vi "FocalMainWakeStudyV3.vi"() -> ()   [LabVIEW 2018]
uses:
  Clusters/FileDataChannel.ctl
  Clusters/BladePitchMode.ctl
  Clusters/GenMode.ctl
  Clusters/IndicatorScale.ctl
  Clusters/SimulationConstants.ctl
  Clusters/PLCTravSignals.ctl
  Clusters/IOSignals.ctl
  <vilib>/Platform/TimedLoop/XDataNode/timing_clust.ctl
  <vilib>/Platform/TimedLoop/XDataNode/nitl_modes.ctl
  <vilib>/Platform/TimedLoop/XDataNode/wakeup.ctl
  Clusters/ArrayPairs.ctl
  Clusters/SwapArrayCluster.ctl
  Clusters/ElmoState.ctl
  Clusters/CtrlSignals.ctl
  Clusters/ScalingEnum.ctl
  Clusters/AnemometerData.ctl
  Clusters/RoscoParams.ctl
  Clusters/GenCtrl.ctl
  Clusters/PitchCtrl.ctl
  <vilib>/Instr/_visa.llb/VISA Configure Serial Port (Instr).vi
  SubVIs/InsertIntoArray_v2.vi
  <vilib>/platform/TimedLoop/XDataNode/XDataNode.xnode
  <vilib>/Platform/TimedLoop/XDataNode/XDNodeRunTimeDep.lvlib
  <resource>/objmgr/IndComECAT.rc
  usr/local/lib/libCallROSCO.so
  <vilib>/ptbypt/NI_PtbyPt.lvlib
panel:
  out "anemoXprobeD2_m_s":dbl
  out "anemoXprobeD1_m_s":dbl
  out "anemoXprobeC2_m_s":dbl
  out "anemoXprobeC1_m_s":dbl
  out "traversePosZ_mm":dbl
  out "traversePosY_mm":dbl
  out "traversePosX_mm":dbl
  in  "PLCTravSignals":T1
  out "WE ROSCO":dbl
  out "Mz":dbl format="%#_5g"
  out "My":dbl format="%#_5g"
  out "Mx":dbl format="%#_5g"
  in  "zeroRotorPos":bool
  out "Fz":dbl format="%#_5g"
  out "TSR":dbl
  out "anemoRefU_m_s":dbl
  out "RS232 loop late?":bool
  in  "Fan Setpoint (%)":dbl format="%#_13g"
  out "Setpoint file loaded":path
  in  "Ctrl Mode":enum32{"Manual", "FromFile"}(radio)
  in  "Setpoint file name":string="setpointsVelTestA.txt"
  in  "Reload File":bool
  in  "windSpeed_m_s":dbl format="%#_13g"
  out "towerBotMy":dbl
  out "Current Setting":dbl[](array[numeric])
  in  "Commit":bool
  in  "Clear Faults":bool
  in  "Enable Fans":bool
  in  "Turn Fans On":bool
  out "Fy":dbl format="%#_5g"
  out "Fx":dbl
  out "PLC read errors":string
  out "PLC read/write late?":bool
  out "PLC Read Error":bool
  out "Axis 3 Homing":bool
  out "Axis 2 Homing":bool
  out "Axis 1 Homing":bool
  in  "Home Blades (x3)":bool
  out "Axis 3 Homed":bool
  out "Axis 2 Homed":bool
  out "Axis 1 Homed":bool
  out "SimulationConst":T2={"nGear"=1.0, "rotorRadius"=120.0, "numBlades"=3, "scaleFactor"=70.0, "roscoInitMinSpeed_rad_s"=0.5, "roscoInitMinTorqueFS_Nm"=1000000.0, "beckhoff16bit"=1000000.0, "beckhoff24BitExt"=7812500, "BX824Bit"=0, "rotorTorqueScale_Nm_V"=5.0, "rotorTorqueOfst_Nm"=2.0, "rangeEL3104V"=10.0, "nacelleAccELM3604V"=1.25, "nacelleAccScaleX_m_s2_V"=0.0673, "nacelleAccOfstX_m_s2"=0.0055, "nacelleAccScaleY_m_s2_V"=0.0672, "nacelleAccOfstY_m_s2"=0.0049, "nacelleAccScaleZ_m_s2_V"=0.0677, "nacelleAccOfstZ_m_s2"=0.0087, "cyberGearRatio"=0.5, "cyberLinesPerRev"=0.5, "cyberRatedTorque"=0.5, "towerTopForceScale"=0.5, "towerTopTorqueScale"=0.5, "plcSetpointScaling_norm2VFD"=0.5, "towerBotScaleMy_Nm_V"=0.5, "towerBotOfstMy_Nm"=0.5, "towerTopScaleXaxis_N_V"=0.5, "towerTopOfstXaxis_N"=0.5, "towerTopScaleYaxis_N_V"=0.5, "towerTopOfstYaxis_N"=0.5, "pitchFlagOffset_deg"=0.5, "anemWindSpeedScaleU_m_s_m_s"=0.5, "anemWindSpeedOfstU_m_s"=0.5, "anemWindSpeedScaleV_m_s_m_s"=0.5, "anemWindSpeedOfstV_m_s"=0.5, "anemWindSpeedScaleW_m_s_m_s"=0.5, "anemWindSpeedOfstW_m_s"=0.5, "anemWindSpeedScaleTSI1_m_s_V"=0.5, "anemWindSpeedOfstTSI1_m_s"=0.5, "anemWindSpeedScaleTSI3_m_s_V"=0.5, "anemWindSpeedOfstTSI3_m_s"=0.5, "anemWindSpeedScaleXProbeA1C0"=0.5, "anemWindSpeedScaleXProbeA1C1"=0.5, "anemWindSpeedScaleXProbeA1C2"=0.5, "anemWindSpeedScaleXProbeA1C3"=0.5, "anemWindSpeedScaleXProbeA1C4"=0.5, "anemWindSpeedOfstXProbeA1_m_s"=0.5, "anemWindSpeedScaleXProbeA2C0"=0.5, "anemWindSpeedScaleXProbeA2C1"=0.5, "anemWindSpeedScaleXProbeA2C2"=0.5, "anemWindSpeedScaleXProbeA2C3"=0.5, "anemWindSpeedScaleXProbeA2C4"=0.5, "anemWindSpeedOfstXProbeA2_m_s"=0.5, "anemWindSpeedScaleXProbeC1C0"=0.5, "anemWindSpeedScaleXProbeC1C1"=0.5, "anemWindSpeedScaleXProbeC1C2"=0.5, "anemWindSpeedScaleXProbeC1C3"=0.5, "anemWindSpeedScaleXProbeC1C4"=0.5, "anemWindSpeedOfstXProbeC1_m_s"=0.5, "anemWindSpeedScaleXProbeC2C0"=0.5, "anemWindSpeedScaleXProbeC2C1"=0.5, "anemWindSpeedScaleXProbeC2C2"=0.5, "anemWindSpeedScaleXProbeC2C3"=0.5, "anemWindSpeedScaleXProbeC2C4"=0.5, "anemWindSpeedOfstXProbeC2_m_s"=0.5, "anemWindSpeedScaleXProbeD1C0"=0.5, "anemWindSpeedScaleXProbeD1C1"=0.5, "anemWindSpeedScaleXProbeD1C2"=0.5, "anemWindSpeedScaleXProbeD1C3"=0.5, "anemWindSpeedScaleXProbeD1C4"=0.5, "anemWindSpeedOfstXProbeD1_m_s"=0.5, "anemWindSpeedScaleXProbeD2C0"=0.5, "anemWindSpeedScaleXProbeD2C1"=0.5, "anemWindSpeedScaleXProbeD2C2"=0.5, "anemWindSpeedScaleXProbeD2C3"=0.5, "anemWindSpeedScaleXProbeD2C4"=0.5, "anemWindSpeedOfstXProbeD2_m_s"=0.5, "anemWindSpeedOfstHw3_m_s"=0.5, "anemWindSpeedScaleHw3_m_s_V"=0.5, "probeAOfstX_mm"=0.5, "probeAOfstY_mm"=0.5, "probeAOfstZ_mm"=0.5, "probeTSIOfstX_mm"=0.5, "probeTSIOfstY_mm"=0.5, "probeTSIOfstZ_mm"=0.5, "probeBOfstX_mm"=0.5, "probeBOfstY_mm"=0.5, "probeBOfstZ_mm"=0.5} {"beckhoff16bit" format="%x"}
  out "nacelleAccZ (m/s2)":dbl
  out "nacelleAccY (m/s2)":dbl
  out "nacelleAccX (m/s2)":dbl
  out "Disk > 2GB free?":bool
  out "Current OP mode":T3
  in  "IndicatorScale":T4
  in  "DISCON.IN file":string="IEA15MW_FOCAL_04_DISCON.IN"
  in  "Cp/Ct/Cq file":string="IEA15MW_FOCAL_00_Cp_Ct_Cq.txt"
  out "Torque sine period FS (Nm)":dbl format="%.2g"
  out "Torque sine amp FS (Nm)":dbl format="%.2g"
  out "Torque sine mean FS (Nm)":dbl format="%.2g"
  out "Ramp time FS (s)":dbl format="%.2g"
  out "Ramp target vel FS (rpm)":dbl format="%.2g"
  out "Const. vel setpoint FS (rpm)":dbl format="%.2g"
  out "From File RotSpd FS (rpm)":dbl
  out "From File Pitch FS (deg)":dbl
  out "Exp time FS (s)":dbl format="%5.2f"
  in  "Commit gen settings":bool
  out "Current OP mode":T5
  in  "Commit pitch settings":bool
  in  "Start / Stop Run":bool
  out "Speed Setpoint (rpm)":dbl(knob)=7.068579725455493e-05 scale=0.0..20.0
  out "Pitch Blade 3 (deg)":dbl
  out "Pitch Bade 2 (deg)":dbl
  out "Pitch Blade 1 (deg)":dbl
  out "Pitch Setpoint (deg)":dbl
  out "Torque sine period MS (Nm)":dbl format="%.2g"
  out "Torque sine amp MS (Nm)":dbl format="%#.2g"
  in  "Torque sine period (s)":dbl=100.0
  in  "Torque sine amp (MNm)":dbl
  out "Torque sine mean MS (Nm)":dbl format="%.2g"
  in  "Torque mean (MNm)":dbl
  out "Ramp time MS (s)":dbl format="%.2g"
  out "Ramp target vel MS (rpm)":dbl format="%.2g"
  out "Const. vel setpoint MS (rpm)":dbl format="%.2g"
  in  "Ramp time (s)":dbl=100.0
  in  "Ramp target vel (rpm)":dbl=1.0
  in  "Const. vel (rpm)":dbl
  out "Current Const. (deg)":dbl
  in  "Next OP mode":T3
  in  "Next Const. (deg)":dbl=10.0
  in  "Next OP mode":T5
  in  "Wind Est. u(t=0)":dbl=5.0
  out "Exp. Time MS (s)":dbl format="%5.1f"
  out "Output file Name":string
  out "State logic late?":bool
  out "Axis 3 Fault":bool
  out "Axis 3 Warning":bool
  out "Axis 2 Fault":bool
  out "Axis 2 Warning":bool
  out "Axis 1 Fault":bool
  out "Axis 1 Warning":bool
  out "Axis 3 Operational":bool
  out "Axis 2 Operational":bool
  out "Axis 1 Operational":bool
  out "Pitch Axis 3 State":string
  out "Pitch Axis 2 State":string
  out "Pitch Axis 1 State":string
  in  "Clear Pitch Actuator Faults (x3)":bool
  in  "Enable Pitch Actuators (x3)":bool
  out "Generator Operational":bool
  in  "Clear Accelnet Faults":bool
  in  "Enable Accelnet":bool
  out "Generator Fault":bool
  out "Generator Warning":bool
  out "Main generator state":string
  out "Rosco Failed?":bool
  out "Torque Cell":dbl(knob) scale=0.0..25.0
  out "Actual Speed MS (rpm)":dbl(knob)=7.068579725455493e-05 scale=0.0..20.0
  in  "?":T6(tab)
  out "Generator Speed":dynamicdata(graph)
  out "Rotor Loads":dynamicdata(graph)
  out "Pitch":dynamicdata(graph)
  in  "Sample":bool
  in  "Apply Ofst":bool
  out "FxMean":dbl format="%0.2f"
  out "FyMean":dbl format="%0.2f"
  out "FzMean":dbl format="%0.2f"
  out "MxMean":dbl format="%0.2f"
  out "MyMean":dbl format="%0.2f"
  out "MzMean":dbl format="%0.2f"
  out "botMyMean":dbl format="%0.2f"
  out "pitch1_deg":dbl
  out "pitch2_deg":dbl
  out "pitch3_deg":dbl
  in  "pitch1 Ofst (deg)":dbl
  in  "pitch3 Ofst (deg)":dbl=-1.5
  in  "pitch2 Ofst (deg)":dbl
  out "Wind":dynamicdata(graph)
  out "DISCON.IN Contents":string
  out "Rosco Interface Current Message":string
  out "ROSCO DISCON.In file used":string
  out "ROSCO CpCqCt File used":string
  out "ROSCO out file used":string
  out "Test sum":sgl
  out "error out":errorcluster
  out "aviFAIL":i32
  out "Rosco Interface First Message":string
  out "Rosco Setpoint (Nm) - MS":dbl(knob) scale=0.0..10.0
  out "OUT_ROTSP":dbl
  out "OUT_AEROTQ":dbl
  out "Rosco Pitch Setpoint (rad)":dbl(knob) scale=0.0..10.0
  out "avrSWAP":dbl[](array[numeric])
  out "Setpoints":dbl[][](array[numeric])
  out "Time index":i32
  out "Loop duration (ms)":i64
  in  "Pitch Max Vel Change (rpm/min) - FS":dbl=10.0
  in  "Pitch Max Vel (rpm) - FS":dbl=1.0
  in  "Pitch Homing Vel  (rpm) - FS":dbl=0.3
  in  "Pitch P-Gain":dbl=5.0
  in  "Max Vel (rpm)  -FS":dbl=14.0
  in  "Velocity Ctrl P-Gain":dbl=0.14
  in  "Velocity Ctrl I-Gain":dbl=3.0
  in  "Torque Ctrl FF Gain":dbl=0.35
  in  "Torque Ctrl I-Gain":dbl=12.5
  in  "Torque Ctrl P-Gain":dbl=0.3
  in  "Max Torque (MNm) - FS":dbl=25.0
  out "Pitch axis 3 ctrl word":u16 format="%x"
  out "Pitch axis 2 ctrl word":u16 format="%x"
  out "RT Loop Duration":i64
  out "Control Mode - Main Gen":u8
  out "WriteSDO Abort - Main Gen":u32
  out "ReadSDO Abort - Main Gen":u32
  out "Gen ctrl word":u16 format="%x"
  out "Pitch axis 1 ctrl word":u16 format="%x"
  out "Graphics Update t (s)":dbl format="%.1f"
  out "Effective graphics rate (ms)":dbl format="%#.1f"
  out "WriteSDO Abort - Pitch 1":u32
  out "ReadSDO Abort - Pitch 1":u32
  out "Control Mode - Pitch 1":u8
  out "Torque RAW (V)":dbl
  out "Torque Sensor (Nm) - NOT scaled":dbl(knob) scale=-2.0..2.0
  out "Free GB disk":dbl
  out "WriteSDO Abort - Pitch 2":u32
  out "Control Mode - Pitch 2":u8
  out "ReadSDO Abort - Pitch 2":u32
  out "WriteSDO Abort - Pitch 3":u32
  out "Control Mode - Pitch 3":u8
  out "ReadSDO Abort - Pitch 3":u32
  out "MotorDemandTorque_Nm":dbl(knob) scale=-2.0..2.0
  out "MotorCurrentTorq (Nm)":dbl(knob) scale=-2.0..2.0
  out "Axis 1 HomePos (rad)":dbl
  out "Axis 2 HomePos (rad)":dbl
  out "Axis 3 HomePos (rad)":dbl
  out "mainGenPosition (deg)":dbl
  out "Init error":errorcluster
  out "Setpoint read error":string
  out "ROSCO Tq Setpoint":dbl(knob) scale=0.0..35.0
  out "Power (MW)":dbl(slide) scale=0.0..30.0 scale format="%.2f"
  out "FIFO Loop Late?":bool
  in  "Base filename":string="rosco-tests"
  out "Writing":bool
  in  "?":T7
  out "#RT FIFO":u32
  in  "Stop LabVIEW":bool
  out "cRio Time(s)":dbl format="%6.1f"
  out "RT Loop Late?":bool
  # "FOCAL Campaign 1 - V2.1"
  # "ROSCO OK?"
  # "GENERATOR ENABLE"
  # "BLADE PITCH"
  # "WIND MACHINE CONTROL"
  # "EXPERIMENT CONTROL"
  # "GENERATOR SETPOINT CTRL"
  # "PITCH ACTUATORS CONTROL"
  # "Nacelle Acceleration"
  # "TowerTop 6DOF"
  # "Blade1"
  # "Blade2"
  # "Blade3"
  # "Current values"
  # "Operational"
  # "Enter NEXT values (FS)"
  # "FS"
  # "MS"
  # "Homing"
  # "Wind Survey"
  # "Homed"
  # "Warning"
  # "Error"
  # "TowerBot My"
  # "Ind Offset, 8/20/2021"
  # "Fan 1"
  # "Time"
  # "Pitch"
  # "RotSpd"
  # "Fan 20"
  # "Fan 30"
  # "Fan 10"
  # "PI for Torque Ctrl"
  # "PI for Velocity Ctrl"
  # "PI for Pitch Ctrl"
  # "Main Gen Limits"
  # "Pitch limits"
  # "PITCH AXIS 1"
  # "PITCH AXIS 2"
  # "PITCH AXIS 3"
  # "TOWER TOP 6DOF"
  # "SYSTEM"
  # "GENERATOR"
  # "TORQUE SENSOR"
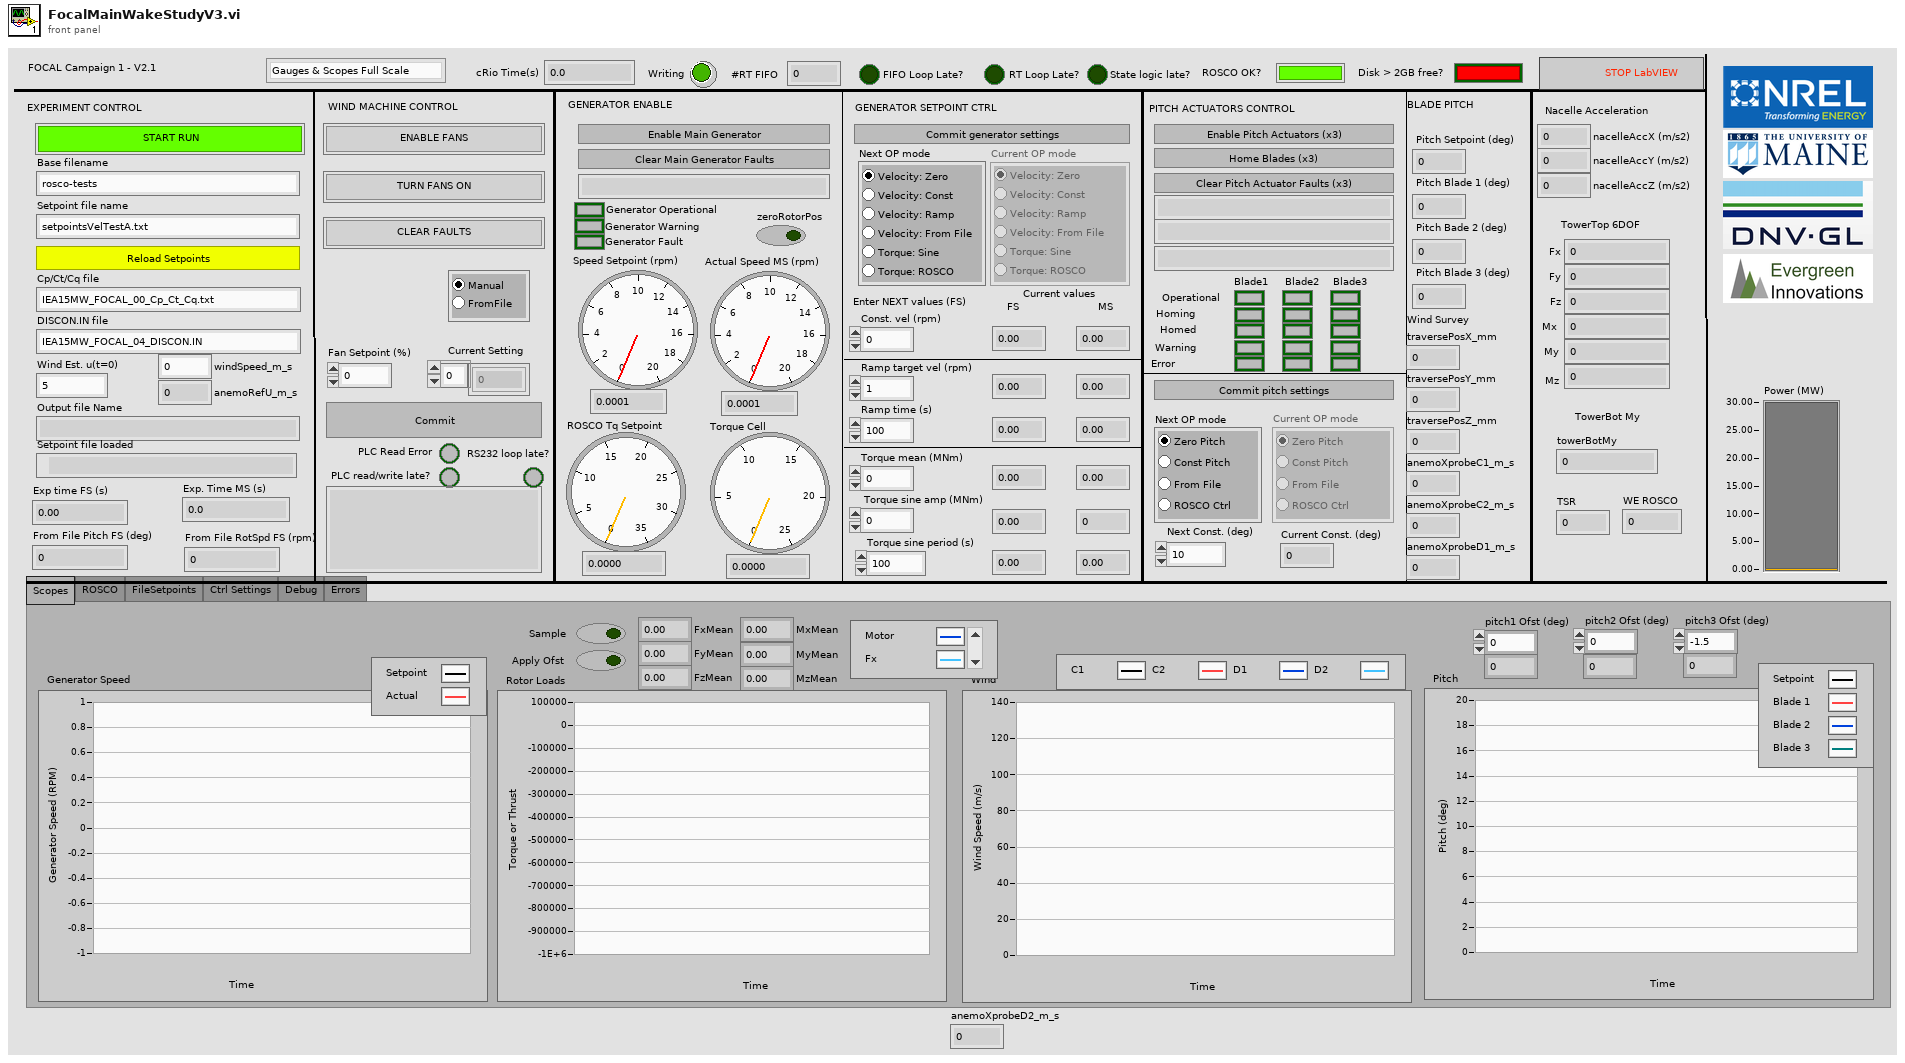
[diagram p1: front panel]
types:
  T1 = typedef "PLCTravSignals.ctl" = cluster{"traversePosX_mm":dbl, "traversePosY_mm":dbl, "traversePosZ_mm":dbl}
  T2 = typedef "SimulationConstants.ctl" = cluster{"nGear":dbl, "rotorRadius":sgl, "numBlades":i32, "scaleFactor":dbl, "roscoInitMinSpeed_rad_s":dbl, "roscoInitMinTorqueFS_Nm":dbl, "beckhoff16bit":dbl, "beckhoff24BitExt":i32, "BX824Bit":i32, "rotorTorqueScale_Nm_V":dbl, "rotorTorqueOfst_Nm":dbl, "rangeEL3104V":dbl, "nacelleAccELM3604V":dbl, "nacelleAccScaleX_m_s2_V":dbl, "nacelleAccOfstX_m_s2":dbl, "nacelleAccScaleY_m_s2_V":dbl, "nacelleAccOfstY_m_s2":dbl, "nacelleAccScaleZ_m_s2_V":dbl, "nacelleAccOfstZ_m_s2":dbl, "cyberGearRatio":dbl, "cyberLinesPerRev":dbl, "cyberRatedTorque":dbl, "towerTopForceScale":dbl, "towerTopTorqueScale":dbl, "plcSetpointScaling_norm2VFD":dbl, "towerBotScaleMy_Nm_V":dbl, "towerBotOfstMy_Nm":dbl, "towerTopScaleXaxis_N_V":dbl, "towerTopOfstXaxis_N":dbl, "towerTopScaleYaxis_N_V":dbl, "towerTopOfstYaxis_N":dbl, "pitchFlagOffset_deg":dbl, "anemWindSpeedScaleU_m_s_m_s":dbl, "anemWindSpeedOfstU_m_s":dbl, "anemWindSpeedScaleV_m_s_m_s":dbl, "anemWindSpeedOfstV_m_s":dbl, "anemWindSpeedScaleW_m_s_m_s":dbl, "anemWindSpeedOfstW_m_s":dbl, "anemWindSpeedScaleTSI1_m_s_V":dbl, "anemWindSpeedOfstTSI1_m_s":dbl, "anemWindSpeedScaleTSI3_m_s_V":dbl, "anemWindSpeedOfstTSI3_m_s":dbl, "anemWindSpeedScaleXProbeA1C0":dbl, "anemWindSpeedScaleXProbeA1C1":dbl, "anemWindSpeedScaleXProbeA1C2":dbl, "anemWindSpeedScaleXProbeA1C3":dbl, "anemWindSpeedScaleXProbeA1C4":dbl, "anemWindSpeedOfstXProbeA1_m_s":dbl, "anemWindSpeedScaleXProbeA2C0":dbl, "anemWindSpeedScaleXProbeA2C1":dbl, "anemWindSpeedScaleXProbeA2C2":dbl, "anemWindSpeedScaleXProbeA2C3":dbl, "anemWindSpeedScaleXProbeA2C4":dbl, "anemWindSpeedOfstXProbeA2_m_s":dbl, "anemWindSpeedScaleXProbeC1C0":dbl, "anemWindSpeedScaleXProbeC1C1":dbl, "anemWindSpeedScaleXProbeC1C2":dbl, "anemWindSpeedScaleXProbeC1C3":dbl, "anemWindSpeedScaleXProbeC1C4":dbl, "anemWindSpeedOfstXProbeC1_m_s":dbl, "anemWindSpeedScaleXProbeC2C0":dbl, "anemWindSpeedScaleXProbeC2C1":dbl, "anemWindSpeedScaleXProbeC2C2":dbl, "anemWindSpeedScaleXProbeC2C3":dbl, "anemWindSpeedScaleXProbeC2C4":dbl, "anemWindSpeedOfstXProbeC2_m_s":dbl, "anemWindSpeedScaleXProbeD1C0":dbl, "anemWindSpeedScaleXProbeD1C1":dbl, "anemWindSpeedScaleXProbeD1C2":dbl, "anemWindSpeedScaleXProbeD1C3":dbl, "anemWindSpeedScaleXProbeD1C4":dbl, "anemWindSpeedOfstXProbeD1_m_s":dbl, "anemWindSpeedScaleXProbeD2C0":dbl, "anemWindSpeedScaleXProbeD2C1":dbl, "anemWindSpeedScaleXProbeD2C2":dbl, "anemWindSpeedScaleXProbeD2C3":dbl, "anemWindSpeedScaleXProbeD2C4":dbl, "anemWindSpeedOfstXProbeD2_m_s":dbl, "anemWindSpeedOfstHw3_m_s":dbl, "anemWindSpeedScaleHw3_m_s_V":dbl, "probeAOfstX_mm":dbl, "probeAOfstY_mm":dbl, "probeAOfstZ_mm":dbl, "probeTSIOfstX_mm":dbl, "probeTSIOfstY_mm":dbl, "probeTSIOfstZ_mm":dbl, "probeBOfstX_mm":dbl, "probeBOfstY_mm":dbl, "probeBOfstZ_mm":dbl}
  T3 = typedef "GenMode.ctl" = enum32{"Velocity: Zero", "Velocity: Const.", "Velocity: Ramp", "Velocity: From File", "Torque: Sine", "Torque: ROSCO"}
  T4 = typedef "IndicatorScale.ctl" = enum16{"Gauges & Scopes Full Scale", "Gauges & Scopes Model Scale"}
  T5 = typedef "BladePitchMode.ctl" = enum32{"Zero pitch", "Const pitch", "From File", "ROSCO Ctrl"}
  T6 = enum32{"Scopes", "ROSCO", "FileSetpoints", "Ctrl Settings", "Debug", "Errors"}
  T7 = typedef "FileDataChannel.ctl" = cluster{"dataTime_s":dbl, "dataLoopCounter":dbl, "anemoRefU_m_s":dbl, "anemoRefV_m_s":dbl, "anemoRefW_m_s":dbl, "rotorTorque_Nm":dbl, "towerTopFx_N":dbl, "towerTopFy_N":dbl, "towerBotMy_Nm":dbl, "accelNacelleAx_m_s2":dbl, "accelNacelleAy_m_s2":dbl, "accelNacelleAz_m_s2":dbl, "genSpeed_rad_s":dbl, "genTorque_Nm":dbl, "genStatus":dbl, "pitch1Position_rad":dbl, "pitch1Velocity_rad_s":dbl, "pitch1Status":dbl, "pitch2Position_rad":dbl, "pitch2Velocity_rad_s":dbl, "pitch2Status":dbl, "pitch3Position_rad":dbl, "pitch3Velocity_rad_s":dbl, "pitch3Status":dbl, "genUserOpMode":dbl, "pitchUserOpMode":dbl, "torqueSetpointRosco_Nm":dbl, "pitchSetpointRosco_rad":dbl, "fan1Setpt_%":dbl, "genTorqueSetpointActual_Nm":dbl, "pitchSetpointActual_rad":dbl, "genVelSetpoint_radps":dbl, "genPosition_rad":dbl, "towerTopFz_N":dbl, "towerTopMx_Nm":dbl, "towerTopMy_Nm":dbl, "towerTopMz_Nm":dbl, "anemoTSIcalU_m_s":dbl, "roscoWE_m_s":dbl, "anemoXprobeA1_m_s":dbl, "anemoXprobeA2_m_s":dbl, "anemoXprobeC1_m_s":dbl, "anemoXprobeC2_m_s":dbl, "anemoXprobeD1_m_s":dbl, "anemoXprobeD2_m_s":dbl, "traversePosX_mm":dbl, "traversePosY_mm":dbl, "traversePosZ_mm":dbl, "probeAPosX_mm":dbl, "probeAPosY_mm":dbl, "probeAPosZ_mm":dbl, "probeCPosX_mm":dbl, "probeCPosY_mm":dbl, "probeCPosZ_mm":dbl, "probeDPosX_mm":dbl, "probeDPosY_mm":dbl, "probeDPosZ_mm":dbl}
  T8 = typedef "CtrlSignals.ctl" = cluster{"Enable":bool, "On":bool, "Reset Fault":bool}
  T9 = typedef "ElmoState.ctl" = cluster{"Elmo Operational":bool, "Elmo Warning":bool, "Elmo Fault":bool, "Blade Homed":bool, "Blade Homing":bool, "HomePos (rad)":dbl}
  T10 = typedef "ArrayPairs.ctl" = cluster{"iStatus":T11, "TIME":T11, "DT":T11, "Blade1PitchPos_rad":T11, "VS_MECHGENPWR":T11, "VS_GENPWR":T11, "GEN_SPEED":T11, "ROTOR_SPEED":T11, "GENTQMEAS":T11, "Y_M":T11, "HORWINDV":T11, "ROOTMOOP1":T11, "ROOTMOOP2":T11, "Blade2PitchPos_rad":T11, "Blade3PitchPos_rad":T11, "ROOTMOOP3":T11, "AVCMSG_SIZE":T11, "INFILE_SIZE ":T11, "OUTFILE_SIZE ":T11, "FA_ACC":T11, "NUM_BLADES":T11, "BladePitchSetpoint_rad":T11, "TorqueSetpoint_Nm":T11, "OUT_AEROTQ":T11, "Out.RotSpeed ":T11, "Out.DEBUG":T11}
  T11 = typedef "SwapArrayCluster.ctl" = cluster{"Index":i32, "Value":dbl}
  T12 = typedef "IOSignals.ctl" = cluster{"mainGenPosition (rad)":dbl, "motorCurrentTorq (Nm)":dbl, "mainGenVelocity (rad/s)":dbl, "mainGenStatus":u16, "pitch1Position (rad)":dbl, "pitch1Velocity (rad/s)":dbl, "pitch1Status":u16, "pitch2Position (rad)":dbl, "pitch2Velocity (rad/s)":dbl, "pitch2Status":u16, "pitch3Position (rad)":dbl, "pitch3Velocity (rad/s)":dbl, "pitch3Status":u16, "torqueSensor (Nm)":dbl, "nacelleAccX (m/s2)":dbl, "nacelleAccY (m/s2)":dbl, "nacelleAccZ (m/s2)":dbl, "pitch1HomeFlag":bool, "pitch2HomeFlag":bool, "pitch3HomeFlag":bool, "towerTopFx (N)":dbl, "towerTopFy (N)":dbl, "towerTopFz (N)":dbl, "towerBotMy (Nm)":dbl, "anemoRefU_m_s":dbl, "anemoRefV_m_s":dbl, "anemoRefW_m_s":dbl, "atiFx_N":dbl, "atiFy_N":dbl, "atiFz_N":dbl, "atiMx_Nm":dbl, "atiMy_Nm":dbl, "atiMz_Nm":dbl, "anemoCalU_m_s":dbl, "anemoXprobeA1_m_s":dbl, "anemoXprobeA2_m_s":dbl, "anemoXprobeC1_m_s":dbl, "anemoXprobeC2_m_s":dbl, "anemoXprobeD1_m_s":dbl, "anemoXprobeD2_m_s":dbl}
  T13 = enum16{"open", "replace", "create", "open or create", "replace or create", "replace or create with confirmation"}
  T14 = typedef "RoscoParams.ctl" = cluster{"avrSWAP":dbl[], "aviFAIL":i32, "currentMsg":string, "ReturnValue":i32, "disconInFileName":string, "outFileName":string, "firstMsg":string}
  T15 = typedef "XDNodeRunTimeDep.lvlib/timing_clust.ctl" = cluster{"Expected End [f-1]":u64, "Actual End [f-1]":u64, "Finished Late? [f-1]":bool, "Expected End [i-1]":u64, "Actual End [i-1]":u64, "Finished Late? [i-1]":bool, "Expected Start [i]":u64, "Actual Start [i]":u64, "Expected Start [f]":u64, "Actual Start [f]":u64, "Source Name":string, "Structure Name":string, "Period":i64, "Deadline":i64, "Offset":i64, "Start":i64, "Priority":i32, "Timeout":i32, "Mode":T16, "Wakeup Reason":T17, "Error":errorcluster, "Source Type":string, "Secondary Source Type":string, "Global End Time":u64, "Global Start Time":u64, "Frame Duration":u64, "Iteration Duration":u64, "Assigned CPU":i32, "I/O Scan Engine Mode":u32}
  T16 = typedef "XDNodeRunTimeDep.lvlib/nitl_modes.ctl" = enum32{"No Change", "Process missed periods, maintain original phase", "Discard missed periods, maintain original phase", "Process missed periods, ignore original phase", "Discard missed periods, ignore original phase"}
  T17 = typedef "XDNodeRunTimeDep.lvlib/wakeup.ctl" = enum32{"Normal", "Aborted", "Asynchronous wakeup", "Timing source error", "Timed loop error", "Timeout"}
  T18 = enum8{"Enabled", "Disabled", "Disabled and Grayed Out"}
  T19 = typedef "ScalingEnum.ctl" = enum16{"Model scale -> Full scale", "Full scale -> Model scale"}
  T20 = typedef "GenCtrl.ctl" = cluster{"Constant velocity setpoint (rpm)":dbl, "Ramp target velocity (rpm)":dbl, "Ramp time (s)":dbl, "Sine mean (Nm)":dbl, "Sine amp (Nm)":dbl, "Sine period (s)":dbl, "Torque Ctrl I-Gain":dbl, "Velocity Ctrl P-Gain":dbl, "Velocity Ctrl I-Gain":dbl, "Max Torque (Nm)":dbl, "GeneratorOn":bool, "Torque Ctrl P-Gain":dbl, "From file velocity (rpm)":dbl, "Generator operating mode":T3, "Max Vel (rpm)":dbl, "Torque Ctrl FF Gain":dbl}
  T21 = typedef "PitchCtrl.ctl" = cluster{"P-Gain":dbl, "Blade pitch operating mode":T5, "Constant setpoint (deg)":dbl, "I-Gain":dbl, "Pitch from File (deg)":dbl, "Homing vel (rpm)":dbl, "Max vel (rpm)":dbl, "Max vel change (rpm/min)":dbl}
  T22 = typedef "AnemometerData.ctl" = cluster{"Wind speed, U (m/s)":dbl, "Wind speed, V (m/s)":dbl, "Wind speed, W (m/s)":dbl}
  T23 = typedef "AccelnetState.ctl" = cluster{"State String":string, "Accelnet Warning":bool, "Accelnet Fault":bool, "Accelnet Operational":bool}
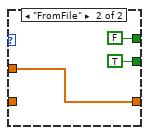
[diagram p6: hidden frame]
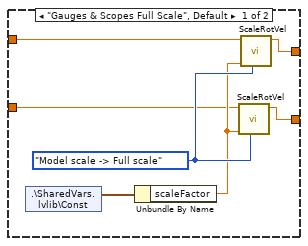
[diagram p11: hidden frame]
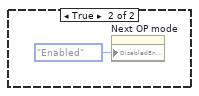
[diagram p14: hidden frame]
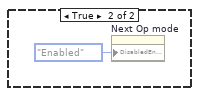
[diagram p15: hidden frame]
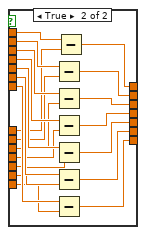
[diagram p17: hidden frame]
diagram:
  w2 = T8 {"Enable"=FALSE, "On"=FALSE, "Reset Fault"=FALSE}  # Ctrl State
  w10 = T8 {"Enable"=FALSE, "On"=FALSE, "Reset Fault"=FALSE}  # Current State
  w8 = errorcluster {"status"=FALSE, "code"=0, "source"=""}  # Error
  w20 = u16 10 items=["1.0"=10, "1.5"=15, "2.0"=20] ("stop bits (10: 1 bit)")
  w21 = u16 0 items=["None", "XON/XOFF", "RTS/CTS", "XON/XOFF & RTS/CTS", "DTR/DSR", "XON/XOFF & DTR/DSR"] ("flow control (0:none)")
  w74 = i64 2000 ("Period")
  # "Setpoint VFD"
  # "Current VFD read from PLC"
  # "Adjust this once we get a feeling for IO latency to/from the PLC"
  # "Run at 62 Hz = 31.25ms = 32150 us"
  # "Manual Vel Set"
  # "Rotor Spd init"
  # "Blade Pitch init"
  # "Velocity Setpoint init"
  # "Time init"
  # "us -> s"
  # "in us"
  # "Init torque sine period"
  # "Init torque sine amp"
  # "Init torque mean"
  # "Init Ramp time"
  # "Init Ramp target vel"
  # "Init Const. Vel"
  # "Initial pitch"
  # "Code to remove"
  # "dt (s)"
  # "5ms = 200Hz"
  # "group name"
  n1 = flat-sequence {
    tunnel: [w123] -> w89
    tunnel: [w124] -> w88
    tunnel: [w116] -> w82
    tunnel: [w115] -> w81
    tunnel: [w102] -> w54
    tunnel: [w101] -> w53
    tunnel: [w100] -> w52
    tunnel: [w99] -> w51
    tunnel: w89 -> [w167]
    tunnel: w88 -> [w166]
    tunnel: w82 -> [w157]
    tunnel: w81 -> [w156]
    tunnel: [w153] -> w48
    tunnel: w54 -> [w144]
    tunnel: w53 -> [w143]
    tunnel: w52 -> [w133]
    tunnel: w51 -> [w132]
    tunnel: w48 -> [w177]
    tunnel: [w177] -> w47
    tunnel: [w225] -> w84
    tunnel: [w219] -> w92
    tunnel: [w212] -> w67
    tunnel: w47 -> [w212]
    tunnel: [w193] -> w56
    frame #0 {
      w100 = refnum<k21> "ni.var.io://NI-cRIO-9036-01B82934/EtherCAT Master/PitchBlade3" ("Slave Constant")
      w102 = refnum<k21> "ni.var.io://NI-cRIO-9036-01B82934/EtherCAT Master/PitchBlade2" ("Slave Constant")
      w116 = refnum<k21> "ni.var.io://NI-cRIO-9036-01B82934/EtherCAT Master/PitchBlade1" ("Slave Constant")
      w123 = refnum<k21> "ni.var.io://NI-cRIO-9036-01B82934/EtherCAT Master/MainGen" ("Slave Constant")
      # "Mode of operation for Pitch Blade 3"
      # "Mode of operation"
      # "8 = CSP \n9 = CSV\n10 = CST"
      # "Mode of operation for Pitch Blade 2"
      # "Mode of operation"
      # "8 = CSP \n9 = CSV\n10 = CST"
      # "Note: Operate in CST, and close velocity loop in LabVIEW when required"
      # "Mode of operation for Pitch Blade 1"
      # "Mode of operation for Main Gen"
      # "Mode of operation"
      # "8 = CSP \n9 = CSV\n10 = CST"
      # "Mode of operation"
      # "9 = CSV\n10 = CST"
      # "Set modes of operation for main generator and pitch actuators"
      n2 = invoke class="IndComECAT Slave" method="neLVRefNum_Slave_WriteSDO"(reference=w116, "Blocking"=TRUE, "OD Addr"=u16 0, "Index"=u16 24672, "Subindex"=u8 0, "Data"=u8[] [9]) -> (error out=w115:errorcluster, "Abort Code"=→"WriteSDO Abort - Pitch 1":u32)  [unwired: 3 in, 7 out]
      n3 = invoke class="IndComECAT Slave" method="neLVRefNum_Slave_WriteSDO"(reference=w102, "Blocking"=TRUE, "OD Addr"=u16 0, "Index"=u16 24672, "Subindex"=u8 0, "Data"=u8[] [9]) -> (error out=w101:errorcluster, "Abort Code"=→"WriteSDO Abort - Pitch 2":u32)  [unwired: 3 in, 7 out]
      n4 = invoke class="IndComECAT Slave" method="neLVRefNum_Slave_WriteSDO"(reference=w123, "Blocking"=TRUE, "OD Addr"=u16 0, "Index"=u16 24672, "Subindex"=u8 0, "Data"=u8[] [10]) -> (error out=w124:errorcluster, "Abort Code"=→"WriteSDO Abort - Main Gen":u32)  [unwired: 3 in, 7 out]
      n5 = invoke class="IndComECAT Slave" method="neLVRefNum_Slave_WriteSDO"(reference=w100, "Blocking"=TRUE, "OD Addr"=u16 0, "Index"=u16 24672, "Subindex"=u8 0, "Data"=u8[] [9]) -> (error out=w99:errorcluster, "Abort Code"=→"WriteSDO Abort - Pitch 3":u32)  [unwired: 3 in, 7 out]
    }
    frame #1 {
      # "Mode of operation"
      # "Mode of operation"
      # "Mode of operation"
      # "Mode of operation"
      # "Check generator and pitch actuator control modes"
      n6 = invoke class="IndComECAT Slave" method="neLVRefNum_Slave_ReadSDO"(reference=w167, error in=w166, "blocking"=TRUE, "odAddr"=u16 0 ("OD address"), "index"=u16 24672 ("Index"), "subIndex"=u8 0 ("Subindex")) -> (error out=w155:errorcluster, "data"=w170:u8[], "abortCode"=→"ReadSDO Abort - Main Gen":u32)  [unwired: 3 in, 6 out]
      n7 = invoke class="IndComECAT Slave" method="neLVRefNum_Slave_ReadSDO"(reference=w144, error in=w143, "blocking"=TRUE, "odAddr"=u16 0 ("OD address"), "index"=u16 24672 ("Index"), "subIndex"=u8 0 ("Subindex")) -> (error out=w142:errorcluster, "data"=w150:u8[], "abortCode"=→"ReadSDO Abort - Pitch 2":u32)  [unwired: 3 in, 6 out]
      n8 = invoke class="IndComECAT Slave" method="neLVRefNum_Slave_ReadSDO"(reference=w133, error in=w132, "blocking"=TRUE, "odAddr"=u16 0 ("OD address"), "index"=u16 24672 ("Index"), "subIndex"=u8 0 ("Subindex")) -> (error out=w131:errorcluster, "data"=w136:u8[], "abortCode"=→"ReadSDO Abort - Pitch 3":u32)  [unwired: 3 in, 6 out]
      n9 = invoke class="IndComECAT Slave" method="neLVRefNum_Slave_ReadSDO"(reference=w157, error in=w156, "blocking"=TRUE, "odAddr"=u16 0 ("OD address"), "index"=u16 24672 ("Index"), "subIndex"=u8 0 ("Subindex")) -> (error out=w154:errorcluster, "data"=w160:u8[], "abortCode"=→"ReadSDO Abort - Pitch 1":u32)  [unwired: 3 in, 6 out]
      n10 = Index Array(array=w170, index=0) -> (element=→"Control Mode - Main Gen":u8)
      n11 = Index Array(array=w150, index=0) -> (element=→"Control Mode - Pitch 2":u8)
      n12 = Index Array(array=w136, index=0) -> (element=→"Control Mode - Pitch 3":u8)
      n13 = Index Array(array=w160, index=0) -> (element=→"Control Mode - Pitch 1":u8)
      n14 = Merge Errors(w155, w154, w142, w131) -> (w153:errorcluster)
    }
    frame #2 {
      w176 = T2 {"nGear"=1.0, "rotorRadius"=120.0, "numBlades"=3, "scaleFactor"=70.0, "roscoInitMinSpeed_rad_s"=0.5, "roscoInitMinTorqueFS_Nm"=1000000.0, "beckhoff16bit"=32768.0, "beckhoff24BitExt"=7812500, "BX824Bit"=8388608, "rotorTorqueScale_Nm_V"=1.0, "rotorTorqueOfst_Nm"=-0.02, "rangeEL3104V"=10.0, "nacelleAccELM3604V"=1.25, "nacelleAccScaleX_m_s2_V"=14.859, "nacelleAccOfstX_m_s2"=0.081724, "nacelleAccScaleY_m_s2_V"=14.881, "nacelleAccOfstY_m_s2"=0.072917, "nacelleAccScaleZ_m_s2_V"=14.771, "nacelleAccOfstZ_m_s2"=0.128508, "cyberGearRatio"=64.0, "cyberLinesPerRev"=4096.0, "cyberRatedTorque"=5.1, "towerTopForceScale"=1000000.0, "towerTopTorqueScale"=1000000.0, "plcSetpointScaling_norm2VFD"=6000.0, "towerBotScaleMy_Nm_V"=193147.3, "towerBotOfstMy_Nm"=-0.0109, "towerTopScaleXaxis_N_V"=93217.84, "towerTopOfstXaxis_N"=-1.19319, "towerTopScaleYaxis_N_V"=88458.94, "towerTopOfstYaxis_N"=1.362268, "pitchFlagOffset_deg"=-4.0, "anemWindSpeedScaleU_m_s_m_s"=1.0, "anemWindSpeedOfstU_m_s"=0.0, "anemWindSpeedScaleV_m_s_m_s"=1.0, "anemWindSpeedOfstV_m_s"=0.0, "anemWindSpeedScaleW_m_s_m_s"=1.0, "anemWindSpeedOfstW_m_s"=0.0, "anemWindSpeedScaleTSI1_m_s_V"=1.0, "anemWindSpeedOfstTSI1_m_s"=0.0, "anemWindSpeedScaleTSI3_m_s_V"=1.0, "anemWindSpeedOfstTSI3_m_s"=0.0, "anemWindSpeedScaleXProbeA1C0"=14.52491, "anemWindSpeedScaleXProbeA1C1"=-31.5795, "anemWindSpeedScaleXProbeA1C2"=25.49783, "anemWindSpeedScaleXProbeA1C3"=-9.5465, "anemWindSpeedScaleXProbeA1C4"=1.634486, "anemWindSpeedOfstXProbeA1_m_s"=0.0, "anemWindSpeedScaleXProbeA2C0"=14.87181, "anemWindSpeedScaleXProbeA2C1"=-30.9244, "anemWindSpeedScaleXProbeA2C2"=24.65621, "anemWindSpeedScaleXProbeA2C3"=-9.62302, "anemWindSpeedScaleXProbeA2C4"=1.752811, "anemWindSpeedOfstXProbeA2_m_s"=0.0, "anemWindSpeedScaleXProbeC1C0"=28.767853, "anemWindSpeedScaleXProbeC1C1"=-68.689629, "anemWindSpeedScaleXProbeC1C2"=62.018379, "anemWindSpeedScaleXProbeC1C3"=-25.983692, "anemWindSpeedScaleXProbeC1C4"=4.521054, "anemWindSpeedOfstXProbeC1_m_s"=0.0, "anemWindSpeedScaleXProbeC2C0"=4.329403, "anemWindSpeedScaleXProbeC2C1"=-11.51335, "anemWindSpeedScaleXProbeC2C2"=11.959132, "anemWindSpeedScaleXProbeC2C3"=-6.54513, "anemWindSpeedScaleXProbeC2C4"=1.731069, "anemWindSpeedOfstXProbeC2_m_s"=0.0, "anemWindSpeedScaleXProbeD1C0"=11.809229, "anemWindSpeedScaleXProbeD1C1"=-27.911182, "anemWindSpeedScaleXProbeD1C2"=25.224531, "anemWindSpeedScaleXProbeD1C3"=-11.088564, "anemWindSpeedScaleXProbeD1C4"=2.202625, "anemWindSpeedOfstXProbeD1_m_s"=0.0, "anemWindSpeedScaleXProbeD2C0"=21.473507, "anemWindSpeedScaleXProbeD2C1"=-47.721043, "anemWindSpeedScaleXProbeD2C2"=40.090096, "anemWindSpeedScaleXProbeD2C3"=-15.906531, "anemWindSpeedScaleXProbeD2C4"=2.758574, "anemWindSpeedOfstXProbeD2_m_s"=0.0, "anemWindSpeedOfstHw3_m_s"=0.0, "anemWindSpeedScaleHw3_m_s_V"=1.0, "probeAOfstX_mm"=0.5, "probeAOfstY_mm"=0.5, "probeAOfstZ_mm"=0.5, "probeTSIOfstX_mm"=0.5, "probeTSIOfstY_mm"=0.5, "probeTSIOfstZ_mm"=0.5, "probeBOfstX_mm"=0.5, "probeBOfstY_mm"=0.5, "probeBOfstZ_mm"=0.5} ("SimulationConst")
      # "Note:\nnacelleAcc constants are inverted (1/x) from manufacturer sheets due to how we apply scale\nConstants are applied based on sensor channel, not basin coordinate system. \nAny change in sign is done in readIO to assign the correct channels and orientation\n\nReference Calibrations_Summary_DATE.xlsx"
      # "Define constants to be used in the code"
      # "Define constants"
      n15 = shared-variable ".\\SharedVars.lvlib\\Const"(w176) -> ()  [unwired: 1 in, 1 out]
      "SimulationConst" <- w176
    }
    frame #3 {
      w205 = path "C:/rosco-data" ("path")
      # "Updated\n2021/09/21"
      # "This file will be picked up via DISCON.IN / ROSCO"
      # "Checks if DISCON.IN exists"
      # "Allocate memory for ROSCO return message"
      # "Up to 500 entries in SWAP array"
      # "No. of buffer slices"
      # "This is the typedef for File IO"
      # "number of channels"
      # "Read required files and initialize various arrays"
      n16 = disable-structure shown="Disabled" {
        frame Disabled {
          # "Note: DO NOT run this code in normal operation. Will  cause the .so file to not unload properly."
          # "Test function into libCallROSCO"
          n17 = dll-call lib="usr/local/lib/libCallROSCO.so" fn="add"("a"=sgl 1.0, "b"=sgl 8.0) -> (error out=→"error out":errorcluster, "sum"=→"Test sum":sgl)  [unwired: 5 in, 1 out]
        }
        frame Enabled {
        }
      }
      n18 = property on="Base filename" class="Str"("Value"="focal_series_000" ("Base filename")) -> ()  [unwired: 2 in, 2 out]
      n19 = property on="Rosco Interface Current Message" class="Str"("Value"="") -> ()  [unwired: 2 in, 2 out]
      n20 = property on="Base filename" class="Str"("Value"="") -> ()  [unwired: 2 in, 2 out]
      n21 = property on="StopLabVIEW" class="Bool (strict)"("Value"=FALSE) -> ()  [unwired: 2 in, 2 out]
      n22 = property on="Enable Accelnet" class="Bool (strict)"("Value"=FALSE ("Enable Accelnet")) -> ()  [unwired: 2 in, 2 out]
      n23 = property on="Enable Pitch Actuators (x3)" class="Bool (strict)"("Value"=FALSE ("Enable Pitch Actuators (x3)")) -> ()  [unwired: 2 in, 2 out]
      n24 = property on="Next Op mode" class="RadioBtnsControl (strict)"("Value"=GenMode."Velocity: Zero" ("Next Op mode")) -> ()  [unwired: 2 in, 2 out]
      n25 = property on="Next OP mode" class="RadioBtnsControl (strict)"("Value"=BladePitchMode."Zero pitch" ("Next OP mode")) -> ()  [unwired: 2 in, 2 out]
      n26 = Build Path(base path=w205, name or relative path="roscoOut.txt") -> (appended path=w203:path)
      n27 = Build Path(base path=w205, name or relative path="Cp/Ct/Cq file") -> (appended path=w210:path)
      n28 = Build Path(base path=w205, name or relative path="DISCON.IN file") -> (appended path=w206:path)
      n29 = call "ConfigFileExists.vi"("Path   In"=w206) -> ("Path Out"=w199:path)  [unwired: 9 in, 1 out]
      n30 = call "ConfigFileExists.vi"("Path   In"=w210) -> ("Path Out"=w209:path)  [unwired: 9 in, 1 out]
      n31 = Path To String(path=w203) -> (string=w202:string)
      "ROSCO out file used" <- w202
      n32 = Path To String(path=w209) -> (string=→"ROSCO CpCqCt File used":string)
      n33 = Path To String(path=w199) -> (string=w201:string)
      "ROSCO DISCON.In file used" <- w201
      n34 = Open/Create/Replace File(file path (use dialog)=w199, operation (0:open)=T13."open") -> (refnum out=w197:refnum<file>, error out=w200:errorcluster)  [unwired: 4 in, 1 out]
      n35 = property on="Velocity Ctrl P-Gain" class="DigNum (strict)"("Value"=0.05 ("Velocity Ctrl P-Gain")) -> ()  [unwired: 2 in, 2 out]
      n36 = property on="Velocity Ctrl I-Gain" class="DigNum (strict)"("Value"=7.0 ("Velocity Ctrl I-Gain")) -> ()  [unwired: 2 in, 2 out]
      n37 = property on="Max Torque (MNm) - FS" class="DigNum (strict)"("Value"=25.0 ("Max Torque (MNm) - FS")) -> ()  [unwired: 2 in, 2 out]
      n38 = property on="Max Vel (rpm)  -FS" class="DigNum (strict)"("Value"=15.0 ("Max Vel (rpm)  -FS")) -> ()  [unwired: 2 in, 2 out]
      n39 = property on="Torque Ctrl P-Gain" class="DigNum (strict)"("Value"=0.3 ("Torque Ctrl P-Gain")) -> ()  [unwired: 2 in, 2 out]
      n40 = property on="Torque Ctrl I-Gain" class="DigNum (strict)"("Value"=12.5 ("Torque Ctrl I-Gain")) -> ()  [unwired: 2 in, 2 out]
      n41 = property on="Torque Ctrl FF Gain" class="DigNum (strict)"("Value"=0.35 ("Torque Ctrl FF Gain")) -> ()  [unwired: 2 in, 2 out]
      n42 = call "StringInit.vi"("accOUTNAME"="First Msg", "dimension size"=8192) -> ("result string"=w189:string)  [unwired: 9 in]
      n43 = call "StringInit.vi"("accOUTNAME"="Current Msg", "dimension size"=8192) -> ("result string"=w192:string)  [unwired: 9 in]
      n44 = Initialize Array(0.0 ("element"), 500 ("dimension size")) -> (w217:dbl[])
      n45 = Read from Text File(file (use dialog)=w197, error in=w200) -> (refnum out=w195:refnum<file>, text=→"DISCON.IN Contents":string, error out=w194:errorcluster)  [unwired: 2 in, 1 out]
      n46 = Close File(refnum=w195, error in=w194) -> (error out=w193:errorcluster)  [unwired: 1 out]
      n47 = Bundle By Name(cluster=T14 {"avrSWAP"=[], "aviFAIL"=0, "currentMsg"="", "ReturnValue"=0, "disconInFileName"="", "outFileName"="", "firstMsg"=""}, "avrSWAP"=w217, "aviFAIL"=-100, "currentMsg"=w192, "firstMsg"=w189, "outFileName"=w202, "disconInFileName"=w201) -> (w219:T14)
      n48 = Cluster To Array(cluster="?") -> (array=w215:dbl[])
      n49 = Array Size(array=w215) -> (size(s)=w214:i32)
      n50 = To Unsigned Long Integer(number=w214) -> (unsigned 32bit integer=w213:u32)
      n51 = RT FIFO Create(0:"DataBuffer" ("name (unnamed)"), 1:dbl[] [] ("appended array"), 4:u32 200, 6:w213) -> (8:w225:refnum<k33>)  [unwired: 4 in, 2 out]
    }
  }
  n52 = disable-structure shown="Disabled" {
    frame Disabled {
      n53 = shared-variable ".\\SharedVars.lvlib\\SIM-GenSpeed_rad_s"(0.009999999776482582 ("RotorSpeed(rad/s)")) -> ()  [unwired: 1 in, 1 out]
      n54 = shared-variable ".\\SharedVars.lvlib\\SIM-BladePitch_rad"(0.0 ("ecat-BladePitch")) -> ()  [unwired: 1 in, 1 out]
      n55 = shared-variable ".\\SharedVars.lvlib\\SIM-WindSpeed_m_s"(0.0 ("WindSpeedSim")) -> ()  [unwired: 1 in, 1 out]
    }
    frame Enabled {
    }
  }
  n56 = disable-structure shown="Disabled" {
    frame Disabled {
      n57 = local read "DISCON.IN Contents"() -> ()  [unwired: 1 in]
    }
    frame Enabled {
    }
  }
  n58 = Merge Errors(w56, w67) -> (→"Init error":errorcluster)
  n59 = property on="SimulationConst" class="Clust (strict)"() -> ("Controls[]"=w46:refnum<vi>[])  [unwired: 2 in, 2 out]
  n60 = for {
    tunnel: w46 -> [w243] mode=indexing
    tunnel: [w244] -> w50 mode=indexing
    tunnel: [w240] -> w49 mode=indexing
    n61 = property class="Ctl"(reference=w243) -> ("Value"=w242:variant)  [unwired: 1 in, 2 out]
    n62 = property class="Ctl"(reference=w243) -> ("Label.Text"=w244:string)  [unwired: 1 in, 2 out]
    n63 = Variant To Data(type=0.0, Variant=w242) -> (data=w240:dbl)  [unwired: 1 in, 1 out]
  }
  n64 = Tick Count (ms)() -> (millisecond timer value=w83:u32)
  n65 = property class="Clust (strict)"() -> ("Controls[]"=w98:refnum<vi>[])  [unwired: 2 in, 2 out]
  n66 = To Double Precision Float(number=w74) -> (double precision float=w73:dbl)
  n67 = call-poly "VISA Configure Serial Port"("VISA resource name"=refnum<visa-resource-name> "ASRL1::INSTR", "timeout (10sec)"=u32 1000, "baud rate (9600)"=u32 38400, "data bits (8)"=u16 8, "parity (0:none)"=enum16{"None", "Odd", "Even", "Mark", "Space"}."None", "stop bits (10: 1 bit)"=w20, "flow control (0:none)"=w21) -> ("VISA resource name out"=w17:refnum<visa-resource-name>, "error out"=w16:errorcluster)  [unwired: 7 in]
  n68 = for {
    tunnel: w98 -> [w246] mode=indexing
    tunnel: [w245] -> w97 mode=indexing
    n69 = property class="Ctl"(reference=w246) -> ("Label.Text"=w245:string)  [unwired: 1 in, 2 out]
  }
  n70 = Divide(x=w73, y=1000000.0) -> (x/y=w72:dbl)
  n71 = Initialize Array(0, 32 ("dimension size")) -> (w5:i32[])
  n72 = Initialize Array(0, 32 ("dimension size")) -> (w1:i32[])
  n73 = VISA Clear(VISA resource name=w17, error in (no error)=w16) -> (VISA resource name out=w15:refnum<visa-resource-name>, error out=w14:errorcluster)
  n74 = Initialize Array(0.0 ("element"), 1 ("dimension size")) -> (w33:dbl[])
  n75 = Initialize Array(0.0 ("element"), 1 ("dimension size")) -> (w30:dbl[])
  n76 = Initialize Array(0.0 ("element"), 1 ("dimension size")) -> (w32:dbl[])
  n77 = Initialize Array(0.0 ("element"), 0 ("dimension size"), 32 ("dimension size")) -> (w31:dbl[][])
  n78 = Initialize Array(0.0 ("element"), 32 ("dimension size")) -> (w27:dbl[])
  n79 = node-c288(i64 50 ("Period")) -> (w71:T15)  [unwired: 3 in]
  n80 = while {
    tunnel: w83 -> [w413]
    i -> [w407]
    stop <- w421 stop-if-true
    w270 = -5.0 ("upper limit")
    w272 = 5.0 ("upper limit")
    w277 = 120.0
    w298 = 0.0
    w330 = ScalingEnum."Model scale -> Full scale" ("Scale Dir")
    # "Blade position\nRelies on rotor enc\nbeing \"zero\" at pitch3"
    # "Disabled due to resource use"
    # "Manually enter wind speed for now"
    # "Note: This WE is NOT available in the standard version of ROSCO. Need to add in ROSCO src code."
    # "TSR = r * omega / u"
    # "MN x rad/s -> MW"
    # "Note: At e.g. 250ms, a chart history of 500 points equates to 20 of real time"
    # "Display/Graphics Loop (non-RT)"
    n81 = shared-variable ".\\SharedVars.lvlib\\IOSignals"() -> (w256:T12)  [unwired: 1 in, 1 out]
    n82 = shared-variable ".\\SharedVars.lvlib\\PitchAxis1State"() -> (w346:T9)  [unwired: 1 in, 1 out]
    n83 = shared-variable ".\\SharedVars.lvlib\\PitchAxis2State"() -> (w339:T9)  [unwired: 1 in, 1 out]
    n84 = shared-variable ".\\SharedVars.lvlib\\PitchAxis3State"() -> (w332:T9)  [unwired: 1 in, 1 out]
    n85 = shared-variable ".\\SharedVars.lvlib\\GenCtrlFS"() -> (w387:T20)  [unwired: 1 in, 1 out]
    n86 = shared-variable ".\\SharedVars.lvlib\\GenCtrlMS"() -> (w402:T20)  [unwired: 1 in, 1 out]
    n87 = shared-variable ".\\SharedVars.lvlib\\RoscoPairs"() -> (w415:T10)  [unwired: 1 in, 1 out]
    n88 = shared-variable ".\\SharedVars.lvlib\\RoscoParams"() -> (w269:T14)  [unwired: 1 in, 1 out]
    n89 = shared-variable ".\\SharedVars.lvlib\\PitchCtrlMS"() -> (w404:T21)  [unwired: 1 in, 1 out]
    n90 = Tick Count (ms)() -> (millisecond timer value=w414:u32)
    n91 = disable-structure shown="Disabled" {
      frame Disabled {
        # "bytes -> Gb"
        # "TODO - MAKE THIS AND + HOME"
        n92 = Get Volume Info(11:path "C:/" ("path")) -> (2:w444:i64)  [unwired: 1 in, 5 out]
        n93 = To Double Precision Float(number=w444) -> (double precision float=w443:dbl)
        n94 = Divide(x=w443, y=1073741824.0) -> (x/y=w441:dbl)
        "Free GB disk" <- w441
        n95 = Greater?(x=w441, y=2.0) -> (0:→"Disk > 2GB free?":bool)
      }
      frame Enabled {
      }
    }
    n96 = Wait (ms)(milliseconds to wait=u32 250 ("Period")) -> ()  [unwired: 1 out]
    n97 = Subtract(x=w414, y=w413) -> (x-y=w410:u32)
    n98 = To Double Precision Float(number=w407) -> (double precision float=w408:dbl)
    n99 = To Double Precision Float(number=w410) -> (double precision float=w409:dbl)
    n100 = Unbundle By Name(w256) -> ("mainGenVelocity (rad/s)"=w356:dbl)
    n101 = shared-variable ".\\SharedVars.lvlib\\MotorDemandTorque_Nm"() -> (→"MotorDemandTorque_Nm":dbl)  [unwired: 1 in, 1 out]
    n102 = Unbundle By Name(w256) -> ("motorCurrentTorq (Nm)"=w369:dbl, "torqueSensor (Nm)"=w372:dbl)
    "Torque Sensor (Nm) - NOT scaled" <- w372
    "MotorCurrentTorq (Nm)" <- w369
    n103 = Unbundle By Name(w256) -> ("anemoXprobeC1_m_s"=w255:dbl, "anemoXprobeC2_m_s"=w254:dbl, "anemoXprobeD1_m_s"=w253:dbl, "anemoXprobeD2_m_s"=w248:dbl)
    n104 = shared-variable ".\\SharedVars.lvlib\\PitchSetpoint_rad"() -> (w405:dbl)  [unwired: 1 in, 1 out]
    n105 = Unbundle By Name(w256) -> ("mainGenPosition (rad)"=w308:dbl)
    n106 = Unbundle By Name(w256) -> ("pitch1Position (rad)"=w391:dbl, "pitch2Position (rad)"=w390:dbl, "pitch3Position (rad)"=w389:dbl)
    n107 = Unbundle By Name(w256) -> ("anemoRefU_m_s"=→"anemoRefU_m_s":dbl)
    n108 = Unbundle By Name(w256) -> ("mainGenVelocity (rad/s)"=w379:dbl)
    n109 = shared-variable ".\\SharedVars.lvlib\\GenVelocitySetpoint_radps"() -> (w380:dbl)  [unwired: 1 in, 1 out]
    n110 = shared-variable ".\\SharedVars.lvlib\\RoscoParams"() -> (w357:T14)  [unwired: 1 in, 1 out]
    n111 = Unbundle By Name(w256) -> ("nacelleAccX (m/s2)"=w312:dbl, "nacelleAccY (m/s2)"=w311:dbl, "nacelleAccZ (m/s2)"=w310:dbl)
    "nacelleAccX (m/s2)" <- w312
    "nacelleAccY (m/s2)" <- w311
    "nacelleAccZ (m/s2)" <- w310
    n112 = shared-variable ".\\SharedVars.lvlib\\RoscoPairs"() -> (w264:T10)  [unwired: 1 in, 1 out]
    n113 = disable-structure shown="Disabled" {
      frame Disabled {
        n114 = shared-variable ".\\SharedVars.lvlib\\GeneratorOn"() -> (w456:bool)  [unwired: 1 in, 1 out]
        n115 = shared-variable ".\\SharedVars.lvlib\\PitchAxis1State"() -> (w455:T9)  [unwired: 1 in, 1 out]
        n116 = shared-variable ".\\SharedVars.lvlib\\PitchAxis2State"() -> (w454:T9)  [unwired: 1 in, 1 out]
        n117 = shared-variable ".\\SharedVars.lvlib\\PitchAxis3State"() -> (w453:T9)  [unwired: 1 in, 1 out]
        n118 = case shown="False" w456 {
          frame False {
            n119 = property on="Next Op mode" class="RadioBtnsControl (strict)"("DisabledEnum"=T18."Disabled and Grayed Out" ("Disabled")) -> ()  [unwired: 2 in, 2 out]
            n120 = property on="Enable Accelnet" class="Bool (strict)"("Value"=FALSE ("Enable Accelnet")) -> ()  [unwired: 2 in, 2 out]
            n121 = property on="Next OP mode" class="RadioBtnsControl (strict)"("Value"=GenMode."Velocity: Zero" ("Next OP mode")) -> ()  [unwired: 2 in, 2 out]
          }
          frame True {
            n122 = property on="Next Op mode" class="RadioBtnsControl (strict)"("DisabledEnum"=T18."Enabled" ("Disabled")) -> ()  [unwired: 2 in, 2 out]
          }
        }
        n123 = Unbundle By Name(w455) -> ("Elmo Operational"=w452:bool, "Blade Homed"=w451:bool)
        n124 = Unbundle By Name(w454) -> ("Elmo Operational"=w450:bool, "Blade Homed"=w449:bool)
        n125 = Unbundle By Name(w453) -> ("Elmo Operational"=w448:bool, "Blade Homed"=w447:bool)
        n126 = Compound Arithmetic op=AND(w452, w451, w450, w449, w448, w447) -> (w446:bool)
        n127 = case shown="False" w446 {
          frame False {
            n128 = property on="Next OP mode" class="RadioBtnsControl (strict)"("DisabledEnum"=T18."Disabled and Grayed Out" ("Disabled")) -> ()  [unwired: 2 in, 2 out]
          }
          frame True {
            n129 = property on="Next OP mode" class="RadioBtnsControl (strict)"("DisabledEnum"=T18."Enabled" ("Disabled")) -> ()  [unwired: 2 in, 2 out]
          }
        }
      }
      frame Enabled {
      }
    }
    n130 = Unbundle By Name(w256) -> ("atiFx_N"=w325:dbl, "atiFy_N"=w326:dbl, "atiFz_N"=w327:dbl, "atiMx_Nm"=w306:dbl, "atiMy_Nm"=w301:dbl, "atiMz_Nm"=w300:dbl, "towerBotMy (Nm)"=w299:dbl)
    n131 = Unbundle By Name(w415) -> ("BladePitchSetpoint_rad.Value"=→"Rosco Pitch Setpoint (rad)":dbl, "TorqueSetpoint_Nm.Value"=→"Rosco Setpoint (Nm) - MS":dbl, "Out.RotSpeed.Value"=→"OUT_ROTSP":dbl, "OUT_AEROTQ.Value"=→"OUT_AEROTQ":dbl)
    n132 = Divide(x=w409, y=1000.0) -> (x/y=→"Graphics Update t (s)":dbl)
    n133 = Unbundle By Name(w346) -> ("Elmo Operational"=→"Axis 1 Operational":bool, "Elmo Warning"=→"Axis 1 Warning":bool, "Elmo Fault"=→"Axis 1 Fault":bool, "Blade Homing"=→"Axis 1 Homing":bool, "Blade Homed"=→"Axis 1 Homed":bool, "HomePos (rad)"=→"Axis 1 HomePos (rad)":dbl)
    n134 = Unbundle By Name(w339) -> ("Elmo Operational"=→"Axis 2 Operational":bool, "Elmo Warning"=→"Axis 2 Warning":bool, "Elmo Fault"=→"Axis 2 Fault":bool, "Blade Homing"=→"Axis 2 Homing":bool, "Blade Homed"=→"Axis 2 Homed":bool, "HomePos (rad)"=→"Axis 2 HomePos (rad)":dbl)
    n135 = Unbundle By Name(w332) -> ("Elmo Operational"=→"Axis 3 Operational":bool, "Elmo Warning"=→"Axis 3 Warning":bool, "Elmo Fault"=→"Axis 3 Fault":bool, "Blade Homing"=→"Axis 3 Homing":bool, "Blade Homed"=→"Axis 3 Homed":bool, "HomePos (rad)"=→"Axis 3 HomePos (rad)":dbl)
    n136 = Unbundle By Name(w387) -> ("Constant velocity setpoint (rpm)"=→"Const. vel setpoint FS (rpm)":dbl, "Ramp target velocity (rpm)"=→"Ramp target vel FS (rpm)":dbl, "Ramp time (s)"=→"Ramp time FS (s)":dbl, "Sine mean (Nm)"=→"Torque sine mean FS (Nm)":dbl, "Sine amp (Nm)"=→"Torque sine amp FS (Nm)":dbl, "Sine period (s)"=→"Torque sine period FS (Nm)":dbl)
    n137 = Unbundle By Name(w269) -> ("avrSWAP"=→"avrSWAP":dbl[], "aviFAIL"=→"aviFAIL":i32, "currentMsg"=→"Rosco Interface Current Message":string, "firstMsg"=→"Rosco Interface First Message":string)
    n138 = Divide(x=w409, y=w408) -> (x/y=→"Effective graphics rate (ms)":dbl)
    n139 = Unbundle By Name(w402) -> ("Generator operating mode"=→"Current OP mode":T3, "Constant velocity setpoint (rpm)"=→"Const. vel setpoint MS (rpm)":dbl, "Ramp target velocity (rpm)"=→"Ramp target vel MS (rpm)":dbl, "Ramp time (s)"=→"Ramp time MS (s)":dbl, "Sine mean (Nm)"=→"Torque sine mean MS (Nm)":dbl, "Sine amp (Nm)"=→"Torque sine amp MS (Nm)":dbl, "Sine period (s)"=→"Torque sine period MS (Nm)":dbl)
    n140 = Unbundle By Name(w404) -> ("Constant setpoint (deg)"=→"Current Const. (deg)":dbl, "Blade pitch operating mode"=→"Current OP mode":T5)
    n141 = shared-variable ".\\SharedVars.lvlib\\Const"() -> (w360:T2)  [unwired: 1 in, 1 out]
    n142 = Unbundle By Name(w357) -> ("avrSWAP"=w355:dbl[])
    n143 = Unbundle By Name(w264) -> ("TorqueSetpoint_Nm.Value"=w263:dbl)
    n144 = Unbundle By Name(w360) -> ("rotorRadius"=w359:sgl, "scaleFactor"=w329:dbl)
    n145 = call "RadToDeg.vi"("rad"=w391) -> ("deg"=w376:dbl)
    "Pitch Blade 1 (deg)" <- w376
    n146 = call "RadToDeg.vi"("rad"=w390) -> ("deg"=w375:dbl)
    "Pitch Bade 2 (deg)" <- w375
    n147 = call "RadToDeg.vi"("rad"=w389) -> ("deg"=w374:dbl)
    "Pitch Blade 3 (deg)" <- w374
    n148 = call "RadToDeg.vi"("rad"=w405) -> ("deg"=w394:dbl)
    "Pitch Setpoint (deg)" <- w394
    n149 = Index Array(array=w355, index=199) -> (element=w262:dbl)
    "WE ROSCO" <- w262
    n150 = call "RadToDeg.vi"("rad"=w308) -> ("deg"=w279:dbl)
    "mainGenPosition (deg)" <- w279
    n151 = Quotient & Remainder(x=w279, y=360.0) -> (x-y*floor(x/y)=w276:dbl, floor(x/y)=w275:dbl)
    n152 = Subtract(x=w276, y=w275) -> (x-y=w273:dbl)
    "pitch3_deg" <- w273
    n153 = case shown="\"Gauges & Scopes Model Scale\"" "IndicatorScale" {
      tunnel: w380 -> [w424 w429]
      tunnel: w379 -> [w425 w430]
      tunnel: [w423 w430] -> w365
      tunnel: [w422 w429] -> w377
      frame "Gauges & Scopes Full Scale", Default {
        w428 = ScalingEnum."Model scale -> Full scale" ("Scale Dir")
        n154 = shared-variable ".\\SharedVars.lvlib\\Const"() -> (w427:T2)  [unwired: 1 in, 1 out]
        n155 = Unbundle By Name(w427) -> ("scaleFactor"=w426:dbl)
        n156 = call "ScaleRotVel.vi"("Scale Dir"=w428, "Scale factor"=w426, "Rotational Velocity (In)"=w424) -> ("Rotational Velocity (Out)"=w422:dbl)  [unwired: 8 in]
        n157 = call "ScaleRotVel.vi"("Scale Dir"=w428, "Scale factor"=w426, "Rotational Velocity (In)"=w425) -> ("Rotational Velocity (Out)"=w423:dbl)  [unwired: 8 in]
      }
      frame "Gauges & Scopes Model Scale" {
      }
    }
    n158 = Subtract(x=w273, y=w277) -> (x-y=w274:dbl)
    "pitch2_deg" <- w274
    n159 = Merge Signals(w394, w376, w375, w374) -> (→"Pitch":dynamicdata)
    n160 = Subtract(x=w274, y=w277) -> (x-y=w271:dbl)
    "pitch1_deg" <- w271
    n161 = Merge Signals(w312, w311, w310) -> ()  [unwired: 1 out]
    n162 = feedback #1(w298) -> (w317:dbl)
    "FxMean" <- w317
    n163 = feedback #2(w298) -> (w287:dbl)
    "FyMean" <- w287
    n164 = feedback #3(w298) -> (w288:dbl)
    "FzMean" <- w288
    n165 = feedback #4(w298) -> (w305:dbl)
    "MxMean" <- w305
    n166 = feedback #5(w298) -> (w291:dbl)
    "MyMean" <- w291
    n167 = feedback #6(w298) -> (w290:dbl)
    "MzMean" <- w290
    n168 = feedback #7(w298) -> (w289:dbl)
    "botMyMean" <- w289
    n169 = case shown="True" "Sample" {
      selector: "Sample" -> [_ w511]
      tunnel: w327 -> [w502 w517]
      tunnel: w326 -> [w503 w516]
      tunnel: w325 -> [w504 w515]
      tunnel: [w504 w515] -> w323
      tunnel: [w503 w516] -> w322
      tunnel: [w502 w517] -> w321
      tunnel: [w500 w519] -> w319
      tunnel: [w501 w518] -> w320
      tunnel: [w499 w520] -> w318
      tunnel: w317 -> [w501 _]
      tunnel: w287 -> [w500 _]
      tunnel: w288 -> [w499 _]
      tunnel: w305 -> [w498 _]
      tunnel: [w498 w514] -> w307
      tunnel: w306 -> [w497 w513]
      tunnel: [w497 w513] -> w303
      tunnel: [w494 w510] -> w297
      tunnel: [w495 w509] -> w296
      tunnel: [w496 w508] -> w295
      tunnel: w301 -> [w493 w507]
      tunnel: w300 -> [w492 w506]
      tunnel: w299 -> [w491 w505]
      tunnel: w289 -> [w496 _]
      tunnel: w290 -> [w495 _]
      tunnel: w291 -> [w494 _]
      tunnel: [w493 w507] -> w294
      tunnel: [w492 w506] -> w293
      tunnel: [w491 w505] -> w292
      frame False {
      }
      frame True {
        w512 = 100 ("sample length")
        n170 = call <vilib>:"Mean PtByPt.vi"("x"=w515, "sample length"=w512, "initialize"=w511) -> ("mean"=w518:dbl)  [unwired: 1 in, 1 out]
        n171 = call <vilib>:"Mean PtByPt.vi"("x"=w516, "sample length"=w512, "initialize"=w511) -> ("mean"=w519:dbl)  [unwired: 1 in, 1 out]
        n172 = call <vilib>:"Mean PtByPt.vi"("x"=w517, "sample length"=w512, "initialize"=w511) -> ("mean"=w520:dbl)  [unwired: 1 in, 1 out]
        n173 = call <vilib>:"Mean PtByPt.vi"("x"=w513, "sample length"=w512, "initialize"=w511) -> ("mean"=w514:dbl)  [unwired: 1 in, 1 out]
        n174 = call <vilib>:"Mean PtByPt.vi"("x"=w507, "sample length"=w512, "initialize"=w511) -> ("mean"=w510:dbl)  [unwired: 1 in, 1 out]
        n175 = call <vilib>:"Mean PtByPt.vi"("x"=w506, "sample length"=w512, "initialize"=w511) -> ("mean"=w509:dbl)  [unwired: 1 in, 1 out]
        n176 = call <vilib>:"Mean PtByPt.vi"("x"=w505, "sample length"=w512, "initialize"=w511) -> ("mean"=w508:dbl)  [unwired: 1 in, 1 out]
      }
    }
    n177 = feedback-in #1(w320) -> ()
    n178 = feedback-in #2(w319) -> ()
    n179 = feedback-in #3(w318) -> ()
    n180 = feedback-in #4(w307) -> ()
    n181 = feedback-in #5(w297) -> ()
    n182 = feedback-in #6(w296) -> ()
    n183 = feedback-in #7(w295) -> ()
    n184 = In Range and Coerce(upper limit=w272, x=w273, lower limit=w270) -> ()  [unwired: 2 out]
    n185 = To Double Precision Float(number=w359) -> (double precision float=w362:dbl)
    n186 = call "ScaleRotVel.vi"("Scale Dir"=w330, "Scale factor"=w329, "Rotational Velocity (In)"=w356) -> ("Rotational Velocity (Out)"=w354:dbl)  [unwired: 8 in]
    n187 = call "ScaleTime.vi"("Scale Dir"=w330, "Scale factor"=w329) -> ()  [unwired: 9 in, 1 out]
    n188 = In Range and Coerce(upper limit=w272, x=w274, lower limit=w270) -> ()  [unwired: 2 out]
    n189 = In Range and Coerce(upper limit=w272, x=w271, lower limit=w270) -> ()  [unwired: 2 out]
    n190 = case shown="False" "Apply Ofst" {
      tunnel: w323 -> [w469 w480]
      tunnel: w322 -> [w468 w486]
      tunnel: w321 -> [w467 w485]
      tunnel: w317 -> [_ w479]
      tunnel: w287 -> [_ w478]
      tunnel: w288 -> [_ w477]
      tunnel: [w469 w490] -> w316
      tunnel: [w468 w489] -> w315
      tunnel: [w467 w488] -> w314
      tunnel: w305 -> [_ w476]
      tunnel: [w466 w487] -> w304
      tunnel: w303 -> [w466 w484]
      tunnel: w294 -> [w465 w483]
      tunnel: w293 -> [w464 w482]
      tunnel: w292 -> [w463 w481]
      tunnel: w291 -> [_ w475]
      tunnel: w290 -> [_ w474]
      tunnel: w289 -> [_ w473]
      tunnel: [w465 w472] -> w286
      tunnel: [w464 w471] -> w285
      tunnel: [w463 w470] -> w284
      frame False {
      }
      frame True {
        n191 = Subtract(x=w486, y=w478) -> (x-y=w489:dbl)
        n192 = Subtract(x=w485, y=w477) -> (x-y=w488:dbl)
        n193 = Subtract(x=w484, y=w476) -> (x-y=w487:dbl)
        n194 = Subtract(x=w483, y=w475) -> (x-y=w472:dbl)
        n195 = Subtract(x=w482, y=w474) -> (x-y=w471:dbl)
        n196 = Subtract(x=w481, y=w473) -> (x-y=w470:dbl)
        n197 = Subtract(x=w480, y=w479) -> (x-y=w490:dbl)
      }
    }
    n198 = disable-structure shown="Disabled" {
      disable-tunnel: w256 -> [w438 _]
      frame Disabled {
        n199 = Unbundle By Name(w438) -> ("atiFx_N"=w437:dbl, "atiFy_N"=w436:dbl, "atiFz_N"=w435:dbl, "atiMx_Nm"=w434:dbl, "atiMy_Nm"=w433:dbl, "atiMz_Nm"=w432:dbl)
        n200 = Merge Signals(w437, w436, w435, w434, w433, w432) -> (w431:dynamicdata)
      }
      frame Enabled {
      }
    }
    n201 = Multiply(x=w362, y=w354) -> (x*y=w361:dbl)
    n202 = shared-variable ".\\SharedVars.lvlib\\PLCTravSignals"() -> (w260:T1)  [unwired: 1 in, 1 out]
    n203 = Divide(x=w361, y=w262) -> (x/y=→"TSR":dbl)
    n204 = case shown="\"Gauges & Scopes Full Scale\", Default" "IndicatorScale" {
      tunnel: w372 -> [w549 w568]
      tunnel: [w554 w568] -> w366
      tunnel: w263 -> [w548 w567]
      tunnel: [w553 w567] -> w367
      tunnel: w369 -> [w547 w566]
      tunnel: [w545 w566] -> w368
      tunnel: [w544 w565] -> w331
      tunnel: [w543 w564] -> w313
      tunnel: [w542 w559] -> w283
      tunnel: w316 -> [w541 w565]
      tunnel: w315 -> [w540 w564]
      tunnel: w314 -> [w538 w560]
      tunnel: w304 -> [w537 w559]
      tunnel: [w539 w560] -> w302
      tunnel: w286 -> [w536 w563]
      tunnel: w285 -> [w535 w562]
      tunnel: w284 -> [w534 w561]
      tunnel: [w533 w563] -> w282
      tunnel: [w532 w562] -> w281
      tunnel: [w531 w561] -> w280
      tunnel: [w530 w556] -> w252
      tunnel: [w529 w557] -> w251
      tunnel: [w528 w558] -> w250
      tunnel: w255 -> [w527 w558]
      tunnel: w254 -> [w526 w557]
      tunnel: w253 -> [w525 w556]
      tunnel: w248 -> [w522 w555]
      tunnel: [w521 w555] -> w247
      frame "Gauges & Scopes Full Scale", Default {
        w524 = ScalingEnum."Model scale -> Full scale" ("Scale Dir")
        n205 = shared-variable ".\\SharedVars.lvlib\\Const"() -> (w550:T2)  [unwired: 1 in, 1 out]
        n206 = Unbundle By Name(w550) -> ("scaleFactor"=w523:dbl)
        n207 = call "ScaleForce.vi"("Scale Dir"=w524, "Scale factor"=w523, "Force (In)"=w541) -> ("Force (Out)"=w544:dbl)  [unwired: 8 in]
        n208 = call "ScaleForce.vi"("Scale Dir"=w524, "Scale factor"=w523, "Force (In)"=w540) -> ("Force (Out)"=w543:dbl)  [unwired: 8 in]
        n209 = call "ScaleForce.vi"("Scale Dir"=w524, "Scale factor"=w523, "Force (In)"=w538) -> ("Force (Out)"=w539:dbl)  [unwired: 8 in]
        n210 = call "ScaleTorque.vi"("Scale Dir"=w524, "Scale factor"=w523, "Torque (In)"=w537) -> ("Torque (Out)"=w542:dbl)  [unwired: 8 in]
        n211 = call "ScaleTorque.vi"("Scale Dir"=w524, "Scale factor"=w523, "Torque (In)"=w536) -> ("Torque (Out)"=w533:dbl)  [unwired: 8 in]
        n212 = call "ScaleTorque.vi"("Scale Dir"=w524, "Scale factor"=w523, "Torque (In)"=w535) -> ("Torque (Out)"=w532:dbl)  [unwired: 8 in]
        n213 = call "ScaleTorque.vi"("Scale Dir"=w524, "Scale factor"=w523, "Torque (In)"=w534) -> ("Torque (Out)"=w531:dbl)  [unwired: 8 in]
        n214 = call "ScaleVel.vi"("Scale Dir"=w524, "Scale factor"=w523, "Vel (In)"=w527) -> ("Vel OUT (Out)"=w528:dbl)  [unwired: 8 in]
        n215 = call "ScaleVel.vi"("Scale Dir"=w524, "Scale factor"=w523, "Vel (In)"=w526) -> ("Vel OUT (Out)"=w529:dbl)  [unwired: 8 in]
        n216 = call "ScaleVel.vi"("Scale Dir"=w524, "Scale factor"=w523, "Vel (In)"=w525) -> ("Vel OUT (Out)"=w530:dbl)  [unwired: 8 in]
        n217 = call "ScaleVel.vi"("Scale Dir"=w524, "Scale factor"=w523, "Vel (In)"=w522) -> ("Vel OUT (Out)"=w521:dbl)  [unwired: 8 in]
        n218 = call "ScaleTorque.vi"("Scale Dir"=w524, "Scale factor"=w523, "Torque (In)"=w547) -> ("Torque (Out)"=w546:dbl)  [unwired: 8 in]
        n219 = call "ScaleTorque.vi"("Scale Dir"=w524, "Scale factor"=w523, "Torque (In)"=w549) -> ("Torque (Out)"=w552:dbl)  [unwired: 8 in]
        n220 = call "ScaleTorque.vi"("Scale Dir"=w524, "Scale factor"=w523, "Torque (In)"=w548) -> ("Torque (Out)"=w551:dbl)  [unwired: 8 in]
        n221 = call "NumBy1E6.vi"("x"=w546) -> ("Mx"=w545:dbl)
        n222 = call "NumBy1E6.vi"("x"=w552) -> ("Mx"=w554:dbl)
        n223 = call "NumBy1E6.vi"("x"=w551) -> ("Mx"=w553:dbl)
      }
      frame "Gauges & Scopes Model Scale" {
      }
    }
    "ROSCO Tq Setpoint" <- w367
    "Torque Cell" <- w366
    "Fx" <- w331
    "Fy" <- w313
    "towerBotMy" <- w280
    "Fz" <- w302
    "Mx" <- w283
    "My" <- w282
    "Mz" <- w281
    "anemoXprobeC1_m_s" <- w250
    "anemoXprobeC2_m_s" <- w251
    "anemoXprobeD1_m_s" <- w252
    "anemoXprobeD2_m_s" <- w247
    n224 = call "RadpsToRPM.vi"("radps"=w365) -> ("rpm"=w393:dbl)
    "Actual Speed MS (rpm)" <- w393
    n225 = call "RadpsToRPM.vi"("radps"=w377) -> ("rpm"=w378:dbl)
    "Speed Setpoint (rpm)" <- w378
    n226 = Unbundle By Name(w260) -> ("traversePosX_mm"=→"traversePosX_mm":dbl, "traversePosY_mm"=→"traversePosY_mm":dbl, "traversePosZ_mm"=→"traversePosZ_mm":dbl)
    n227 = Compound Arithmetic op=MULTIPLY(w365, w366) -> (→"Power (MW)":dbl)
    n228 = Merge Signals(w378, w393) -> (w392:dynamicdata)
    n229 = Merge Signals(w392) -> (→"Generator Speed":dynamicdata)
    n230 = shared-variable ".\\SharedVars.lvlib\\StopLabVIEW"() -> (w421:bool)  [unwired: 1 in, 1 out]
    n231 = Merge Signals(w367, w366, w368, w331, w313, w302, w283, w282, w281, w280) -> (→"Rotor Loads":dynamicdata)
    n232 = Merge Signals(w250, w251, w252, w247) -> (→"Wind":dynamicdata)
  }
  n233 = node-c288(w74) -> (w80:T15)  [unwired: 3 in]
  n234 = node-c288(i64 200 ("Period")) -> (w12:T15)  [unwired: 3 in]
  n235 = node-c288(i64 32150 ("Period")) -> (w26:T15)  [unwired: 3 in]
  n236 = node-c288(i64 5 ("Period")) -> (w91:T15)  [unwired: 3 in]
  n237 = node-c288(i64 5 ("Period")) -> (w87:T15)  [unwired: 3 in]
  n238 = timed-loop {
    timing: w71 -> [_]
    timing-out: [_] -> w70
    shift-right: [w647] -> _
    shift-left: BladePitchMode."Zero pitch" ("PitchCtrlMode") -> [w664]
    shift-right: [w648] -> _
    shift-left: 0.0 -> [w662]
    shift-right: [w607] -> _
    shift-left: GenMode."Velocity: Zero" ("GenOpMode") -> [w660]
    shift-right: [w623] -> _
    shift-left: 0.0 -> [w633]
    shift-right: [w621] -> _
    shift-left: 5.0 -> [w632]
    shift-right: [w620] -> _
    shift-left: 100.0 -> [w631]
    shift-right: [w616] -> _
    shift-left: 0.0 -> [w630]
    shift-right: [w615] -> _
    shift-left: 0.0 -> [w629]
    shift-right: [w614] -> _
    shift-left: 0.0 -> [w628]
    shift-right: [w592] -> _
    shift-left: w33 -> [w597]
    shift-right: [w588] -> _
    shift-left: w30 -> [w596]
    shift-right: [w587] -> _
    shift-left: w32 -> [w595]
    shift-right: [w578] -> _
    shift-left: w31 -> [w594]
    shift-right: [w574] -> _
    shift-left: w27 -> [w575]
    stop <- w671 stop-if-true
    w618 = 1000000.0 ("y")
    w646 = T20 {"Constant velocity setpoint (rpm)"=0.0, "Ramp target velocity (rpm)"=0.0, "Ramp time (s)"=0.0, "Sine mean (Nm)"=0.0, "Sine amp (Nm)"=0.0, "Sine period (s)"=0.0, "Torque Ctrl I-Gain"=0.0, "Velocity Ctrl P-Gain"=0.0, "Velocity Ctrl I-Gain"=0.0, "Max Torque (Nm)"=0.0, "GeneratorOn"=FALSE, "Torque Ctrl P-Gain"=0.0, "From file velocity (rpm)"=0.0, "Generator operating mode"=enum."Velocity: Zero", "Max Vel (rpm)"=0.0, "Torque Ctrl FF Gain"=0.0}  # Gen Control
    w651 = T21 {"P-Gain"=0.0, "Blade pitch operating mode"=enum."From File", "Constant setpoint (deg)"=0.0, "I-Gain"=0.0, "Pitch from File (deg)"=0.0, "Homing vel (rpm)"=0.0, "Max vel (rpm)"=0.0, "Max vel change (rpm/min)"=0.0}  # PitchCtrl
    # "Probably not required, but leave in cluster if needed"
    # "This code finds the NEAREST LOWER time. For example, if elements 40s and 50s exist in the input time vector, and tnow = 49s, the code will find the index for 40s."
    # "MNm-> Nm"
    # "Scale right after user input"
    # "Scale right after user input"
    # "MNm-> Nm"
    # "File setpoint and mode loop (RT, but only at 50 ms)"
    n239 = node-c288() -> (→"Loop duration (ms)":i64)  [unwired: 1 in]
    n240 = First Call?() -> (First Call?: T/F=w569:bool)
    n241 = Or(x=w569, y="Reload File") -> (x .or. y?=w571:bool)
    n242 = case shown="True" w571 {
      tunnel: "Setpoint file name" -> [_ w710]
      tunnel: [w702 w707] -> w592
      tunnel: [w700 w706] -> w588
      tunnel: [w699 w705] -> w587
      tunnel: [w701 w704] -> w578
      tunnel: w597 -> [w702 _]
      tunnel: w596 -> [w700 _]
      tunnel: w595 -> [w699 _]
      tunnel: w594 -> [w701 _]
      frame False {
      }
      frame True {
        n243 = call "ReadSetpointFile-v2.vi"("Setpoint file name"=w710) -> ("Fan Vel Set"=w704:dbl[][], "Rotor Spd Set"=w705:dbl[], "Pitch Set"=w706:dbl[], "Time"=w707:dbl[], "Setpoint file loaded"=→"Setpoint file loaded":path, "Setpoint indicator"=→"Setpoints":dbl[][], "Read error"=→"Setpoint read error":string)  [unwired: 4 in]
      }
    }
    n244 = shared-variable ".\\SharedVars.lvlib\\ExpTime_s"() -> (w670:dbl)  [unwired: 1 in, 1 out]
    n245 = shared-variable ".\\SharedVars.lvlib\\Const"() -> (w669:T2)  [unwired: 1 in, 1 out]
    n246 = case shown="True" "Commit" {
      tunnel: "Fan Setpoint (%)" -> [_ w716]
      tunnel: w575 -> [w711 _]
      tunnel: [w711 w712] -> w574
      frame False {
      }
      frame True {
        n247 = Initialize Array(1.0 ("element"), 32 ("dimension size")) -> (w713:dbl[])
        n248 = Multiply(x=w716, y=w713) -> (x*y=w712:dbl[])
      }
    }
    n249 = case shown="True" "Commit gen settings" {
      tunnel: w660 -> [w680 _]
      tunnel: [w680 w687] -> w606
      tunnel: "Next OP mode" -> [_ w687]
      tunnel: "Const. vel (rpm)" -> [_ w686]
      tunnel: "Ramp target vel (rpm)" -> [_ w685]
      tunnel: "Ramp time (s)" -> [_ w684]
      tunnel: "Torque mean (MNm)" -> [_ w683]
      tunnel: "Torque sine amp (MNm)" -> [_ w682]
      tunnel: "Torque sine period (s)" -> [_ w681]
      tunnel: w633 -> [w679 _]
      tunnel: w632 -> [w678 _]
      tunnel: w631 -> [w677 _]
      tunnel: w630 -> [w676 _]
      tunnel: w629 -> [w675 _]
      tunnel: w628 -> [w674 _]
      tunnel: [w679 w686] -> w623
      tunnel: [w678 w685] -> w621
      tunnel: [w677 w684] -> w620
      tunnel: [w676 w683] -> w616
      tunnel: [w675 w682] -> w615
      tunnel: [w674 w681] -> w614
      frame False {
      }
      frame True {
      }
    }
    n250 = shared-variable ".\\SharedVars.lvlib\\GeneratorOn"() -> (w608:bool)  [unwired: 1 in, 1 out]
    n251 = Unbundle By Name(w669) -> ("scaleFactor"=w668:dbl)
    n252 = case shown="True" "Commit pitch settings" {
      tunnel: w664 -> [w727 _]
      tunnel: [w727 w729] -> w647
      tunnel: "Next OP mode" -> [_ w729]
      tunnel: w662 -> [w726 _]
      tunnel: [w726 w728] -> w648
      tunnel: "Next Const. (deg)" -> [_ w728]
      frame False {
      }
      frame True {
      }
    }
    n253 = call "ScaleTime.vi"("Scale Dir"=ScalingEnum."Model scale -> Full scale", "Scale factor"=w668, "Time (In)"=w670) -> ("Time OUT (Out)"=w666:dbl)  [unwired: 8 in]
    "Exp time FS (s)" <- w666
    n254 = case shown="False" w608 {
      tunnel: [GenMode."Velocity: Zero" ("Next OP mode") w673] -> w607
      tunnel: w606 -> [_ w673]
      frame False {
      }
      frame True {
      }
    }
    n255 = Subtract(x=w592, y=w666) -> (x-y=w593:dbl[])
    n256 = shared-variable ".\\SharedVars.lvlib\\FromFileVelFS_rpm"() -> (w640:dbl)  [unwired: 1 in, 1 out]
    n257 = shared-variable ".\\SharedVars.lvlib\\GeneratorOn"() -> (w638:bool)  [unwired: 1 in, 1 out]
    n258 = shared-variable ".\\SharedVars.lvlib\\FromFilePitchFS_deg"() -> (w649:dbl)  [unwired: 1 in, 1 out]
    n259 = Array Size(array=w593) -> (size(s)=w610:i32)
    n260 = Less Or Equal To 0?(x=w593) -> (x <= 0?=w611:bool[])
    n261 = for {
      N: w610 -> [_]
      tunnel: w611 -> [w720] mode=indexing
      shift-right: [w717] -> w591
      shift-left: w593 -> [w719]
      i -> [w718]
      n262 = case shown="False" w720 {
        tunnel: w719 -> [w721 w725]
        tunnel: w718 -> [w724 _]
        tunnel: [w722 w725] -> w717
        frame False {
          n263 = Replace Array Subset(array=w721, new element=nan ("new element/subarray"), index=w724) -> (w722:dbl[])
        }
        frame True {
        }
      }
    }
    n264 = Multiply(x=1000000.0 ("y"), y="Max Torque (MNm) - FS") -> (x*y=w644:dbl)
    n265 = Multiply(x=w618, y=w616) -> (x*y=w619:dbl)
    n266 = Multiply(x=w615, y=w618) -> (x*y=w617:dbl)
    n267 = shared-variable ".\\SharedVars.lvlib\\Const"() -> (w604:T2)  [unwired: 1 in, 1 out]
    n268 = shared-variable ".\\SharedVars.lvlib\\Const"() -> (w637:T2)  [unwired: 1 in, 1 out]
    n269 = Bundle By Name(cluster=w651, "Blade pitch operating mode"=w647, "P-Gain"="Pitch P-Gain", "I-Gain"=0.0, "Constant setpoint (deg)"=w648, "Pitch from File (deg)"=w649, "Homing vel (rpm)"="Pitch Homing Vel  (rpm) - FS", "Max vel (rpm)"="Pitch Max Vel (rpm) - FS", "Max vel change (rpm/min)"="Pitch Max Vel Change (rpm/min) - FS") -> (w624:T21)
    n270 = Bundle By Name(cluster=w646, "Sine period (s)"=w614, "Sine amp (Nm)"=w617, "Sine mean (Nm)"=w619, "Ramp time (s)"=w620, "Ramp target velocity (rpm)"=w621, "Constant velocity setpoint (rpm)"=w623, "Generator operating mode"=w607, "GeneratorOn"=w638, "From file velocity (rpm)"=w640, "Max Torque (Nm)"=w644, "Max Vel (rpm)"="Max Vel (rpm)  -FS", "Torque Ctrl P-Gain"="Torque Ctrl P-Gain", "Torque Ctrl I-Gain"="Torque Ctrl I-Gain", "Torque Ctrl FF Gain"="Torque Ctrl FF Gain", "Velocity Ctrl P-Gain"="Velocity Ctrl P-Gain", "Velocity Ctrl I-Gain"="Velocity Ctrl I-Gain") -> (w622:T20)
    n271 = Absolute Value(x=w591) -> (abs(x)=w590:dbl[])
    n272 = Unbundle By Name(w604) -> ("scaleFactor"=w625:dbl)
    n273 = Array Max & Min(array=w590) -> (min index (indices)=w576:i32)  [unwired: 3 out]
    "Time index" <- w576
    n274 = Array Subset(array=w578, index (row)=w576, length (row)=1 ("length")) -> (w577:dbl[][])  [unwired: 2 in]
    n275 = Reshape Array(w577, 32 ("dimension size")) -> (w585:dbl[])
    n276 = case shown="\"Manual\", Default" "Ctrl Mode" {
      tunnel: [TRUE ("ManualOn") FALSE ("ManualOn")] -> _
      tunnel: [FALSE ("ManualOn") TRUE ("ManualOn")] -> _
      tunnel: [w691 w696] -> w581
      tunnel: w585 -> [_ w696]
      tunnel: w574 -> [w692 _]
      frame "Manual", Default {
        # "From % to [0,1]"
        n277 = Divide(x=w692, y=100.0) -> (x/y=w691:dbl[])
      }
      frame "FromFile" {
      }
    }
    n278 = Unbundle By Name(w637) -> ("scaleFactor"=w636:dbl)
    n279 = In Range and Coerce(upper limit=1.0, x=w581, lower limit=0.0) -> (coerced(x)=w573:dbl[])  [unwired: 1 out]
    "Current Setting" <- w573
    n280 = call "ScalePitchCtrl.vi"("Scale Direction"=ScalingEnum."Full scale -> Model scale", "Scale Factor"=w625, "PitchCtrl (In)"=w624) -> ("PitchCtrl (Out)"=w627:T21)  [unwired: 8 in]
    n281 = Index Array(array=w588, index=w576) -> (element=w584:dbl)
    "From File Pitch FS (deg)" <- w584
    n282 = Index Array(array=w587, index=w576) -> (element=w572:dbl)
    "From File RotSpd FS (rpm)" <- w572
    n283 = shared-variable ".\\SharedVars.lvlib\\StopLabVIEW"() -> (w671:bool)  [unwired: 1 in, 1 out]
    n284 = call "ScaleGenCtrl.vi"("Scale Dir"=ScalingEnum."Full scale -> Model scale", "Scale factor"=w636, "Gen Control (In)"=w622) -> ("Gen Control (Out)"=w634:T20)  [unwired: 8 in]
    n285 = shared-variable ".\\SharedVars.lvlib\\PitchCtrlFS"(w624) -> ()  [unwired: 1 in, 1 out]
    n286 = shared-variable ".\\SharedVars.lvlib\\FromFilePitchFS_deg"(w584) -> ()  [unwired: 1 in, 1 out]
    n287 = shared-variable ".\\SharedVars.lvlib\\FromFileVelFS_rpm"(w572) -> ()  [unwired: 1 in, 1 out]
    n288 = shared-variable ".\\SharedVars.lvlib\\FanSetpoint_unit"(w573) -> ()  [unwired: 1 in, 1 out]
    n289 = shared-variable ".\\SharedVars.lvlib\\PitchCtrlMS"(w627) -> ()  [unwired: 1 in, 1 out]
    n290 = shared-variable ".\\SharedVars.lvlib\\GenCtrlFS"(w622) -> ()  [unwired: 1 in, 1 out]
    n291 = shared-variable ".\\SharedVars.lvlib\\GenCtrlMS"(w634) -> ()  [unwired: 1 in, 1 out]
    n292 = node-c288() -> ()  [unwired: 1 in, 1 out]
  }
  n293 = timed-loop {
    timing: w80 -> [_]
    timing-out: [_] -> w79
    shift-right: [w737] -> _
    shift-left: w92 -> [w778]
    shift-right: [w738] -> w77
    shift-left: errorcluster {"status"=FALSE, "code"=0, "source"=""} ("error out") -> [w777]
    shift-right: [w752] -> _
    shift-left: T10 {"iStatus"={"Index"=0, "Value"=0.0}, "TIME"={"Index"=1, "Value"=0.0}, "DT"={"Index"=2, "Value"=0.0}, "Blade1PitchPos_rad"={"Index"=3, "Value"=0.0}, "VS_MECHGENPWR"={"Index"=13, "Value"=0.0}, "VS_GENPWR"={"Index"=14, "Value"=0.0}, "GEN_SPEED"={"Index"=19, "Value"=0.0}, "ROTOR_SPEED"={"Index"=20, "Value"=0.0}, "GENTQMEAS"={"Index"=22, "Value"=0.0}, "Y_M"={"Index"=23, "Value"=0.0}, "HORWINDV"={"Index"=26, "Value"=0.0}, "ROOTMOOP1"={"Index"=29, "Value"=0.0}, "ROOTMOOP2"={"Index"=30, "Value"=0.0}, "Blade2PitchPos_rad"={"Index"=32, "Value"=0.0}, "Blade3PitchPos_rad"={"Index"=33, "Value"=0.0}, "ROOTMOOP3"={"Index"=31, "Value"=0.0}, "AVCMSG_SIZE"={"Index"=48, "Value"=0.0}, "INFILE_SIZE "={"Index"=49, "Value"=0.0}, "OUTFILE_SIZE "={"Index"=50, "Value"=0.0}, "FA_ACC"={"Index"=52, "Value"=0.0}, "NUM_BLADES"={"Index"=60, "Value"=0.0}, "BladePitchSetpoint_rad"={"Index"=44, "Value"=0.0}, "TorqueSetpoint_Nm"={"Index"=46, "Value"=0.0}, "OUT_AEROTQ"={"Index"=91, "Value"=0.0}, "Out.RotSpeed "={"Index"=92, "Value"=0.0}, "Out.DEBUG"={"Index"=93, "Value"=0.0}} ("ArrayPairs") -> [w779]
    shift-right: [w748] -> _
    shift-left: T12 {"mainGenPosition (rad)"=0.0, "motorCurrentTorq (Nm)"=0.0, "mainGenVelocity (rad/s)"=0.0, "mainGenStatus"=0, "pitch1Position (rad)"=0.0, "pitch1Velocity (rad/s)"=0.0, "pitch1Status"=0, "pitch2Position (rad)"=0.0, "pitch2Velocity (rad/s)"=0.0, "pitch2Status"=0, "pitch3Position (rad)"=0.0, "pitch3Velocity (rad/s)"=0.0, "pitch3Status"=0, "torqueSensor (Nm)"=0.0, "nacelleAccX (m/s2)"=0.0, "nacelleAccY (m/s2)"=0.0, "nacelleAccZ (m/s2)"=0.0, "pitch1HomeFlag"=FALSE, "pitch2HomeFlag"=FALSE, "pitch3HomeFlag"=FALSE, "towerTopFx (N)"=0.0, "towerTopFy (N)"=0.0, "towerTopFz (N)"=0.0, "towerBotMy (Nm)"=0.0, "anemoRefU_m_s"=0.0, "anemoRefV_m_s"=0.0, "anemoRefW_m_s"=0.0, "atiFx_N"=0.0, "atiFy_N"=0.0, "atiFz_N"=0.0, "atiMx_Nm"=0.0, "atiMy_Nm"=0.0, "atiMz_Nm"=0.0, "anemoCalU_m_s"=0.0, "anemoXprobeA1_m_s"=0.0, "anemoXprobeA2_m_s"=0.0, "anemoXprobeC1_m_s"=0.0, "anemoXprobeC2_m_s"=0.0, "anemoXprobeD1_m_s"=0.0, "anemoXprobeD2_m_s"=0.0} -> [w776]
    tunnel: w72 -> [w773]
    tunnel: w72 -> [w772]
    i -> [w739]
    stop <- w782 stop-if-true
    # "ADDED TO DEBUG PITCH"
    # "Main/Control/Execution Loop"
    n294 = node-c288() -> (→"RT Loop Late?":bool, →"RT Loop Duration":i64)  [unwired: 1 in]
    n295 = shared-variable ".\\SharedVars.lvlib\\PitchAxis3State"() -> (w740:T9)  [unwired: 1 in, 1 out]
    n296 = shared-variable ".\\SharedVars.lvlib\\PitchAxis2State"() -> (w741:T9)  [unwired: 1 in, 1 out]
    n297 = shared-variable ".\\SharedVars.lvlib\\PitchAxis1State"() -> (w742:T9)  [unwired: 1 in, 1 out]
    n298 = To Double Precision Float(number=w739) -> (double precision float=w774:dbl)
    n299 = call "ReadIO.vi"("ArrayPairs In"=w779, "PitchAxis1State"=w742, "PitchAxis2State"=w741, "PitchAxis3State"=w740, "IO Signals In"=w776, "ROSCO Params In"=w778, "error in"=w777, "zeroRotorPos"="zeroRotorPos") -> ("ArrayPairs Out"=w771:T10, "IO Signals Out"=w768:T12, "ROSCO Params Out"=w770:T14, "Torque RAW (V)"=→"Torque RAW (V)":dbl, "error out"=w769:errorcluster)  [unwired: 3 in]
    n300 = Multiply(x=w774, y=w773) -> (x*y=w747:dbl)
    "cRio Time(s)" <- w747
    n301 = call "AssignStatus_v2.vi"("Time (s)"=w747, "Rosco dt (s)"=w772, "LoopCount"=w739, "Wind Estimator u(t=0) FS"="Wind Est. u(t=0)", "error in (no error)"=w769, "ROSCO Params In"=w770, "IO Signals In"=w768, "ArrayPairs In"=w771) -> ("error out"=w765:errorcluster, "ROSCO Params Out"=w766:T14, "IO Signals Out"=w764:T12, "ArrayPairs Out"=w767:T10)
    n302 = shared-variable ".\\SharedVars.lvlib\\CtrlLoopTime_s"(w747) -> ()  [unwired: 1 in, 1 out]
    n303 = call "CreateSwapArray_v4.vi"("Loop count"=w739, "error in (no error)"=w765, "ROSCO Params"=w766, "IO Signals In"=w764, "ArrayPairs"=w767) -> ("error out"=w760:errorcluster, "ROSCO Params Out"=w761:T14, "IO Signals Out"=w759:T12, "ArrayPairs Out"=w762:T10)  [unwired: 3 in]
    n304 = shared-variable ".\\SharedVars.lvlib\\PitchCtrlMS"() -> (w746:T21)  [unwired: 1 in, 1 out]
    n305 = call "CallRosco_v2.vi"("StopLV"="Stop LabVIEW", "error in (no error)"=w760, "ROSCO Params in"=w761, "IO Signals In"=w759, "ArrayPairs"=w762) -> ("error out"=w758:errorcluster, "ROSCO Params Out"=w743:T14, "IO Signals Out"=w775:T12, "ArrayPairs Out"=w744:T10)  [unwired: 3 in]
    n306 = shared-variable ".\\SharedVars.lvlib\\GenCtrlMS"() -> (w745:T20)  [unwired: 1 in, 1 out]
    n307 = Build Array("pitch1 Ofst (deg)", "pitch2 Ofst (deg)", "pitch3 Ofst (deg)") -> (w731:dbl[])
    n308 = call "PitchCtrl.vi"("ArrayPairs In"=w744, "IO Signals In"=w775, "ROSCO Params in"=w743, "error in (no error)"=w758, "PitchCtrl"=w746, "Time (s)"=w747, "PitchAxis1State"=w742, "pitchOfst"=w731, "PitchAxis2State"=w741, "PitchAxis3State"=w740) -> ("Pitch setpoint (rad)"=w757:dbl, "ArrayPairs Out"=w756:T10, "IO Signals Out"=w755:T12, "ROSCO Params Out"=w754:T14, "error out"=w753:errorcluster)  [unwired: 5 in]
    n309 = shared-variable ".\\SharedVars.lvlib\\PitchSetpoint_rad"(w757) -> ()  [unwired: 1 in, 1 out]
    n310 = call "GenCtrlCst.vi"("Loop Time (s)"=w747, "Gen Control"=w745, "error in (no error)"=w753, "ROSCO Params in"=w754, "IO Signals In"=w755, "ArrayPairs In"=w756) -> ("error out"=w738:errorcluster, "ROSCO Params Out"=w737:T14, "IO Signals Out"=w748:T12, "ArrayPairs Out"=w752:T10, "Velocity setpoint (rad/s)"=w749:dbl, "Torque setpoint (Nm)"=w750:dbl)
    n311 = shared-variable ".\\SharedVars.lvlib\\GenTorqueSetpoint_Nm"(w750) -> ()  [unwired: 1 in, 1 out]
    n312 = shared-variable ".\\SharedVars.lvlib\\GenVelocitySetpoint_radps"(w749) -> ()  [unwired: 1 in, 1 out]
    n313 = Unbundle By Name(w737) -> ("aviFAIL"=w735:i32)
    n314 = shared-variable ".\\SharedVars.lvlib\\RoscoParams"(w737) -> ()  [unwired: 1 in, 1 out]
    n315 = shared-variable ".\\SharedVars.lvlib\\RoscoPairs"(w752) -> ()  [unwired: 1 in, 1 out]
    n316 = Or(x=w738, y="Stop LabVIEW") -> (x .or. y?=w782:bool)
    n317 = shared-variable ".\\SharedVars.lvlib\\IOSignals"(w748) -> ()  [unwired: 1 in, 1 out]
    n318 = Not Equal To 0?(x=w735) -> (x != 0?=→"Rosco Failed?":bool)
    n319 = shared-variable ".\\SharedVars.lvlib\\StopLabVIEW"(w782) -> ()  [unwired: 1 in, 1 out]
    n320 = node-c288() -> ()  [unwired: 1 in, 1 out]
  }
  n321 = timed-loop {
    timing: w12 -> [_]
    timing-out: [_] -> w11
    shift-right: [w817] -> _
    shift-left: w10 -> [w819]
    shift-right: [w800] -> _
    shift-left: w5 -> [w813]
    shift-right: [w799] -> _
    shift-left: w2 -> [w812]
    shift-right: [w794] -> _
    shift-left: w1 -> [w811]
    shift-right: [w818] -> _
    shift-left: w8 -> [w821]
    stop <- w816 stop-if-true
    w793 = "192.168.1.52"  # PLC IP address
    # "192.168.1.52"
    # "Loop to update the PLC read / write tags"
    n322 = node-c288() -> (→"PLC read/write late?":bool)  [unwired: 1 in]
    n323 = disable-structure shown="Disabled" {
      disable-tunnel: w821 -> [w834 _]
      disable-tunnel: [w833 _] -> w820
      disable-tunnel: w819 -> [w832 _]
      disable-tunnel: w793 -> [w831 _]
      disable-tunnel: [w830 _] -> w814
      disable-tunnel: w813 -> [w829 _]
      disable-tunnel: w812 -> [w828 _]
      disable-tunnel: w811 -> [w827 _]
      disable-tunnel: [w826 _] -> w810
      disable-tunnel: [w825 _] -> w809
      disable-tunnel: [w824 _] -> w808
      disable-tunnel: [w823 _] -> w807
      disable-tunnel: [w822 _] -> w806
      frame Disabled {
        n324 = call "ReadPLC.vi"("PLC Current State In"=w832, "PLC IP address"=w831, "PLC Current VFD In"=w829, "PLC Setpoint State In"=w828, "PLC Setpoint VFD In"=w827, "Error In"=w834) -> ("PLC Current State Out"=w826:T8, "PLC Current VFD Out"=w825:i32[], "PLC Setpoint State Out"=w824:T8, "PLC Setpoint VFD Out"=w823:i32[], "Read Error"=w830:bool, "Read errors"=w833:string, "Error Out"=w822:errorcluster)  [unwired: 3 in]
      }
      frame Enabled {
      }
    }
    "PLC read errors" <- w820
    "PLC Read Error" <- w814
    n325 = shared-variable ".\\SharedVars.lvlib\\FanSetpoint_unit"() -> (w798:dbl[])  [unwired: 1 in, 1 out]
    n326 = call "PLCCtrl.vi"("PLC Current State In"=w810, "FanSetpoint_uint"=w798, "PLC Current VFD In"=w809, "PLC Setpoint State In"=w808, "PLC Setpoint VFD In"=w807, "Error In"=w806, "Enable Fans"="Enable Fans", "Turn Fans On"="Turn Fans On", "Clear Faults"="Clear Faults") -> ("PLC Current State Out"=w805:T8, "PLC Current VFD Out"=w804:i32[], "PLC Setpoint State Out"=w803:T8, "PLC Setpoint VFD Out"=w802:i32[], "Error Out"=w801:errorcluster)  [unwired: 2 in]
    n327 = call "WritePLC.vi"("PLC Current State In"=w805, "PLC IP address"=w793, "PLC Current VFD In"=w804, "Ctrl Setpoint State In"=w803, "PLC Setpoint VFD In"=w802, "Error In"=w801) -> ("PLC Current State Out"=w817:T8, "PLC Current VFD Out"=w800:i32[], "PLC Setpoint State Out"=w799:T8, "PLC Setpoint VFD Out"=w794:i32[], "Error Out"=w818:errorcluster)  [unwired: 5 in]
    n328 = call "Traverse_Sub_Read_Position.vi"("Network Path"=w793) -> ("z position mm"=w790:sgl, "y position mm"=w791:sgl, "x position mm"=w792:sgl)  [unwired: 7 in, 1 out]
    n329 = Bundle By Name(cluster="PLCTravSignals", "traversePosX_mm"=w792, "traversePosY_mm"=w791, "traversePosZ_mm"=w790) -> (w789:T1)
    n330 = shared-variable ".\\SharedVars.lvlib\\PLCTravSignals"(w789) -> ()  [unwired: 1 in, 1 out]
    n331 = shared-variable ".\\SharedVars.lvlib\\StopLabVIEW"() -> (w816:bool)  [unwired: 1 in, 1 out]
    n332 = node-c288() -> ()  [unwired: 1 in, 1 out]
  }
  n333 = timed-loop {
    timing: w26 -> [_]
    timing-out: [_] -> w25
    tunnel: w15 -> [w852]
    tunnel: [w852] -> _
    shift-right: [w838] -> _
    shift-left: w14 -> [w851]
    stop <- w848 stop-if-true
    # "Last byte should be \\r"
    # "22 is a full read for 3 channels and EOL /r"
    # "Loop to update the wind data via RS232"
    n334 = node-c288() -> (→"RS232 loop late?":bool)  [unwired: 1 in]
    n335 = VISA Read(VISA resource name=w852, byte count=u32 22, error in (no error)=w851) -> (VISA resource name out=w841:refnum<visa-resource-name>, read buffer=w842:string, error out=w839:errorcluster)  [unwired: 1 out]
    n336 = call "AnemoASCIIConversion.vi"("Input string (from RS232)"=w842) -> ("Data out"=w847:T22)
    n337 = shared-variable ".\\SharedVars.lvlib\\AnemometerData"(w847) -> ()  [unwired: 1 in, 1 out]
    n338 = String To Byte Array(string=w842) -> (unsigned byte array=w845:u8[])
    n339 = Index Array(array=w845, index=21) -> (element=w844:u8)
    n340 = Equal?(x=w844, y=u8 13) -> (x = y?=w840:bool)
    n341 = case shown="False" w840 {
      tunnel: [w855 w858] -> _
      tunnel: w841 -> [w856 w858]
      tunnel: w839 -> [w854 w857]
      tunnel: [w853 w857] -> w838
      frame False {
        # "If not, flush buffer"
        n342 = VISA Clear(VISA resource name=w856, error in (no error)=w854) -> (VISA resource name out=w855:refnum<visa-resource-name>, error out=w853:errorcluster)
      }
      frame True {
      }
    }
    n343 = shared-variable ".\\SharedVars.lvlib\\StopLabVIEW"() -> (w848:bool)  [unwired: 1 in, 1 out]
    n344 = node-c288() -> ()  [unwired: 1 in, 1 out]
  }
  n345 = timed-loop {
    timing: w91 -> [_]
    timing-out: [_] -> w90
    shift-right: [w865] -> _
    shift-left: T9 {"Elmo Operational"=FALSE, "Elmo Warning"=FALSE, "Elmo Fault"=FALSE, "Blade Homed"=FALSE, "Blade Homing"=FALSE, "HomePos (rad)"=0.0} ("Elmo State Cluster In") -> [w873]
    shift-right: [w864] -> _
    shift-left: T9 {"Elmo Operational"=FALSE, "Elmo Warning"=FALSE, "Elmo Fault"=FALSE, "Blade Homed"=FALSE, "Blade Homing"=FALSE, "HomePos (rad)"=0.0} ("Elmo State Cluster In") -> [w871]
    shift-right: [w863] -> _
    shift-left: T9 {"Elmo Operational"=FALSE, "Elmo Warning"=FALSE, "Elmo Fault"=FALSE, "Blade Homed"=FALSE, "Blade Homing"=FALSE, "HomePos (rad)"=0.0} ("Elmo State Cluster In") -> [w869]
    stop <- w890 stop-if-true
    # "TO DO:\nOnly allow home button when OP\nClear homing state when not in OP\nCheck if home pos (zero) remains consitent while drive is on/off and LabVIEW is on/off\nSet setpoint to zero when not homed"
    # "used in ctrl loop"
    # "used in ctrl loop"
    # "used in ctrl loop"
    # "Axis No. 3"
    # "Axis No. 2"
    # "Axis No. 1"
    # "State logic"
    n346 = node-c288() -> (→"State logic late?":bool)  [unwired: 1 in]
    n347 = shared-variable ".\\SharedVars.lvlib\\IOSignals"() -> (w862:T12)  [unwired: 1 in, 1 out]
    n348 = call "AccelnetInterface.vi"("Enable"="Enable Accelnet", "Clear Faults"="Clear Accelnet Faults", "IO Signals"=w862) -> ("Control word"=w885:u16, "Accelnet State"=w889:T23)  [unwired: 7 in]
    "Gen ctrl word" <- w885
    n349 = call "ElmoInterface.vi"("Elmo State Cluster In"=w873, "Axis No."=u32 1, "IO Signals"=w862, "Enable"="Enable Pitch Actuators (x3)", "Clear faults"="Clear Pitch Actuator Faults (x3)", "Home"="Home Blades (x3)") -> ("Elmo State Cluster Out"=w865:T9, "State String"=→"Pitch Axis 1 State":string, "Control word"=w882:u16)  [unwired: 7 in]
    "Pitch axis 1 ctrl word" <- w882
    n350 = call "ElmoInterface.vi"("Elmo State Cluster In"=w871, "Axis No."=u32 2, "IO Signals"=w862, "Enable"="Enable Pitch Actuators (x3)", "Clear faults"="Clear Pitch Actuator Faults (x3)", "Home"="Home Blades (x3)") -> ("Elmo State Cluster Out"=w864:T9, "State String"=→"Pitch Axis 2 State":string, "Control word"=w879:u16)  [unwired: 7 in]
    "Pitch axis 2 ctrl word" <- w879
    n351 = call "ElmoInterface.vi"("Elmo State Cluster In"=w869, "Axis No."=u32 3, "IO Signals"=w862, "Enable"="Enable Pitch Actuators (x3)", "Clear faults"="Clear Pitch Actuator Faults (x3)", "Home"="Home Blades (x3)") -> ("Elmo State Cluster Out"=w863:T9, "State String"=→"Pitch Axis 3 State":string, "Control word"=w878:u16)  [unwired: 7 in]
    "Pitch axis 3 ctrl word" <- w878
    n352 = Unbundle By Name(w889) -> ("State String"=→"Main generator state":string, "Accelnet Warning"=→"Generator Warning":bool, "Accelnet Fault"=→"Generator Fault":bool, "Accelnet Operational"=w880:bool)
    "Generator Operational" <- w880
    n353 = shared-variable "NI-cRIO-9036-01B82934\\EtherCAT Master\\MainGen\\Receive PDO 7 CST-Control word"(w885) -> ()  [unwired: 1 in, 1 out]
    n354 = shared-variable ".\\SharedVars.lvlib\\PitchAxis2State"(w864) -> ()  [unwired: 1 in, 1 out]
    n355 = shared-variable "NI-cRIO-9036-01B82934\\EtherCAT Master\\PitchBlade2\\Outputs-Control word"(w879) -> ()  [unwired: 1 in, 1 out]
    n356 = shared-variable ".\\SharedVars.lvlib\\PitchAxis1State"(w865) -> ()  [unwired: 1 in, 1 out]
    n357 = shared-variable "NI-cRIO-9036-01B82934\\EtherCAT Master\\PitchBlade1\\Outputs-Control word"(w882) -> ()  [unwired: 1 in, 1 out]
    n358 = shared-variable ".\\SharedVars.lvlib\\PitchAxis3State"(w863) -> ()  [unwired: 1 in, 1 out]
    n359 = shared-variable "NI-cRIO-9036-01B82934\\EtherCAT Master\\PitchBlade3\\Outputs-Control word"(w878) -> ()  [unwired: 1 in, 1 out]
    n360 = shared-variable ".\\SharedVars.lvlib\\GeneratorOn"(w880) -> ()  [unwired: 1 in, 1 out]
    n361 = shared-variable ".\\SharedVars.lvlib\\StopLabVIEW"() -> (w890:bool)  [unwired: 1 in, 1 out]
    n362 = node-c288() -> ()  [unwired: 1 in, 1 out]
  }
  n363 = timed-loop {
    timing: w87 -> [_]
    timing-out: [_] -> w86
    tunnel: w84 -> [w961]
    i -> [w956]
    stop <- w962 stop-if-true
    # "ACCEL ZEROED IN ReadIO"
    # "Data recording to RT buffer"
    n364 = node-c288() -> (→"FIFO Loop Late?":bool)  [unwired: 1 in]
    n365 = shared-variable ".\\SharedVars.lvlib\\IOSignals"() -> (w959:T12)  [unwired: 1 in, 1 out]
    n366 = shared-variable ".\\SharedVars.lvlib\\PitchCtrlMS"() -> (w935:T21)  [unwired: 1 in, 1 out]
    n367 = shared-variable ".\\SharedVars.lvlib\\RoscoPairs"() -> (w940:T10)  [unwired: 1 in, 1 out]
    n368 = shared-variable ".\\SharedVars.lvlib\\RoscoParams"() -> (w908:T14)  [unwired: 1 in, 1 out]
    n369 = shared-variable ".\\SharedVars.lvlib\\GenCtrlMS"() -> (w936:T20)  [unwired: 1 in, 1 out]
    n370 = call "FileWriteTiming.vi"("Loop counter"=w956, "WriteData"="Start / Stop Run") -> ("Write counter"=w955:i32, "Time (s)"=w938:dbl)  [unwired: 8 in]
    n371 = shared-variable ".\\SharedVars.lvlib\\WriteData"("Start / Stop Run") -> ()  [unwired: 1 in, 1 out]
    n372 = shared-variable ".\\SharedVars.lvlib\\GenVelocitySetpoint_radps"() -> (w926:dbl)  [unwired: 1 in, 1 out]
    n373 = Unbundle By Name(w908) -> ("avrSWAP"=w907:dbl[])
    n374 = Unbundle By Name(w936) -> ("Generator operating mode"=w934:T3)
    n375 = Unbundle By Name(w940) -> ("TorqueSetpoint_Nm.Value"=w930:dbl, "BladePitchSetpoint_rad.Value"=w929:dbl)  [unwired: 4 out]
    n376 = shared-variable ".\\SharedVars.lvlib\\GenTorqueSetpoint_Nm"() -> (w928:dbl)  [unwired: 1 in, 1 out]
    n377 = Unbundle By Name(w959) -> ("anemoRefU_m_s"=w919:dbl, "anemoCalU_m_s"=w904:dbl, "anemoXprobeA1_m_s"=w903:dbl, "anemoXprobeA2_m_s"=w902:dbl, "anemoXprobeC1_m_s"=w897:dbl, "anemoXprobeC2_m_s"=w896:dbl, "anemoXprobeD1_m_s"=w895:dbl, "anemoXprobeD2_m_s"=w894:dbl, "torqueSensor (Nm)"=w920:dbl, "atiFx_N"=w924:dbl, "atiFy_N"=w923:dbl, "atiFz_N"=w917:dbl, "atiMx_Nm"=w915:dbl, "atiMy_Nm"=w914:dbl, "atiMz_Nm"=w913:dbl, "towerBotMy (Nm)"=w916:dbl, "nacelleAccX (m/s2)"=w912:dbl, "nacelleAccY (m/s2)"=w911:dbl, "nacelleAccZ (m/s2)"=w910:dbl, "mainGenVelocity (rad/s)"=w958:dbl, "motorCurrentTorq (Nm)"=w957:dbl, "mainGenPosition (rad)"=w918:dbl, "mainGenStatus"=w953:u16, "pitch1Position (rad)"=w952:dbl, "pitch1Velocity (rad/s)"=w951:dbl, "pitch1Status"=w949:u16, "pitch2Position (rad)"=w948:dbl, "pitch2Velocity (rad/s)"=w947:dbl, "pitch2Status"=w946:u16, "pitch3Position (rad)"=w944:dbl, "pitch3Velocity (rad/s)"=w943:dbl, "pitch3Status"=w942:u16)
    n378 = Unbundle By Name(w935) -> ("Blade pitch operating mode"=w931:T5)
    n379 = shared-variable ".\\SharedVars.lvlib\\PitchSetpoint_rad"() -> (w927:dbl)  [unwired: 1 in, 1 out]
    n380 = shared-variable ".\\SharedVars.lvlib\\FanSetpoint_unit"() -> (w922:dbl[])  [unwired: 1 in, 1 out]
    n381 = shared-variable ".\\SharedVars.lvlib\\PLCTravSignals"() -> (w901:T1)  [unwired: 1 in, 1 out]
    n382 = Index Array(array=w907, index=199) -> (element=w905:dbl)
    n383 = To Double Precision Float(number=w955) -> (double precision float=w960:dbl)
    n384 = Unbundle By Name(w901) -> ("traversePosX_mm"=w900:dbl, "traversePosZ_mm"=w899:dbl, "traversePosY_mm"=w898:dbl)
    n385 = To Double Precision Float(number=w953) -> (double precision float=w954:dbl)
    n386 = To Double Precision Float(number=w949) -> (double precision float=w950:dbl)
    n387 = To Double Precision Float(number=w946) -> (double precision float=w945:dbl)
    n388 = To Double Precision Float(number=w934) -> (double precision float=w933:dbl)
    n389 = To Double Precision Float(number=w931) -> (double precision float=w932:dbl)
    n390 = To Double Precision Float(number=w942) -> (double precision float=w941:dbl)
    n391 = Index Array(array=w922, index=0) -> (element=w906:dbl)
    n392 = Bundle By Name(cluster=T7 {"dataTime_s"=0.0, "dataLoopCounter"=0.0, "anemoRefU_m_s"=0.0, "anemoRefV_m_s"=0.0, "anemoRefW_m_s"=0.0, "rotorTorque_Nm"=0.0, "towerTopFx_N"=0.0, "towerTopFy_N"=0.0, "towerBotMy_Nm"=0.0, "accelNacelleAx_m_s2"=0.0, "accelNacelleAy_m_s2"=0.0, "accelNacelleAz_m_s2"=0.0, "genSpeed_rad_s"=0.0, "genTorque_Nm"=0.0, "genStatus"=0.0, "pitch1Position_rad"=0.0, "pitch1Velocity_rad_s"=0.0, "pitch1Status"=0.0, "pitch2Position_rad"=0.0, "pitch2Velocity_rad_s"=0.0, "pitch2Status"=0.0, "pitch3Position_rad"=0.0, "pitch3Velocity_rad_s"=0.0, "pitch3Status"=0.0, "genUserOpMode"=0.0, "pitchUserOpMode"=0.0, "torqueSetpointRosco_Nm"=0.0, "pitchSetpointRosco_rad"=0.0, "fan1Setpt_%"=0.0, "genTorqueSetpointActual_Nm"=0.0, "pitchSetpointActual_rad"=0.0, "genVelSetpoint_radps"=0.0, "genPosition_rad"=0.0, "towerTopFz_N"=0.0, "towerTopMx_Nm"=0.0, "towerTopMy_Nm"=0.0, "towerTopMz_Nm"=0.0, "anemoTSIcalU_m_s"=0.0, "roscoWE_m_s"=0.0, "anemoXprobeA1_m_s"=0.0, "anemoXprobeA2_m_s"=0.0, "anemoXprobeC1_m_s"=0.0, "anemoXprobeC2_m_s"=0.0, "anemoXprobeD1_m_s"=0.0, "anemoXprobeD2_m_s"=0.0, "traversePosX_mm"=0.0, "traversePosY_mm"=0.0, "traversePosZ_mm"=0.0, "probeAPosX_mm"=0.0, "probeAPosY_mm"=0.0, "probeAPosZ_mm"=0.0, "probeCPosX_mm"=0.0, "probeCPosY_mm"=0.0, "probeCPosZ_mm"=0.0, "probeDPosX_mm"=0.0, "probeDPosY_mm"=0.0, "probeDPosZ_mm"=0.0} ("SwapIn"), "dataTime_s"=w938, "dataLoopCounter"=w960, "anemoRefU_m_s"=w919, "anemoTSIcalU_m_s"=w904, "anemoXprobeA1_m_s"=w903, "anemoXprobeA2_m_s"=w902, "anemoXprobeC1_m_s"=w897, "anemoXprobeC2_m_s"=w896, "anemoXprobeD1_m_s"=w895, "anemoXprobeD2_m_s"=w894, "rotorTorque_Nm"=w920, "towerTopFx_N"=w924, "towerTopFy_N"=w923, "towerTopFz_N"=w917, "towerTopMx_Nm"=w915, "towerTopMy_Nm"=w914, "towerTopMz_Nm"=w913, "towerBotMy_Nm"=w916, "accelNacelleAx_m_s2"=w912, "accelNacelleAy_m_s2"=w911, "accelNacelleAz_m_s2"=w910, "genSpeed_rad_s"=w958, "genTorque_Nm"=w957, "genPosition_rad"=w918, "genStatus"=w954, "pitch1Position_rad"=w952, "pitch1Velocity_rad_s"=w951, "pitch1Status"=w950, "pitch2Position_rad"=w948, "pitch2Velocity_rad_s"=w947, "pitch2Status"=w945, "pitch3Position_rad"=w944, "pitch3Velocity_rad_s"=w943, "pitch3Status"=w941, "genUserOpMode"=w933, "pitchUserOpMode"=w932, "torqueSetpointRosco_Nm"=w930, "pitchSetpointRosco_rad"=w929, "roscoWE_m_s"=w905, "fan1Setpt_%"=w906, "genTorqueSetpointActual_Nm"=w928, "pitchSetpointActual_rad"=w927, "genVelSetpoint_radps"=w926, "traversePosX_mm"=w900, "traversePosY_mm"=w899, "traversePosZ_mm"=w898) -> (w925:T7)
    n393 = call "FileBuffer.vi"("Write Data"="Start / Stop Run", "FileDataChannel"=w925, "Refnum in"=w961) -> ("dataTime_s"=w937:dbl, "# elements"=→"#RT FIFO":u32)  [unwired: 7 in]
    "Exp. Time MS (s)" <- w937
    n394 = shared-variable ".\\SharedVars.lvlib\\ExpTime_s"(w937) -> ()  [unwired: 1 in, 1 out]
    n395 = shared-variable ".\\SharedVars.lvlib\\StopLabVIEW"() -> (w962:bool)  [unwired: 1 in, 1 out]
    n396 = node-c288() -> ()  [unwired: 1 in, 1 out]
  }
  n397 = while {
    shift-right: [w975] -> _
    shift-left: _ -> [w976]
    shift-right: [w981] -> _
    shift-left: FALSE -> [w982]
    shift-right: [w984] -> w93
    shift-left: errorcluster {"status"=FALSE, "code"=0, "source"=""} ("error out") -> [w983]
    tunnel: "focalC1" -> [w978]
    tunnel: w97 -> [w971]
    tunnel: w84 -> [w979]
    tunnel: w50 -> [w970]
    tunnel: w49 -> [w969]
    stop <- w986 stop-if-true
    # "Access the file system every 200ms, writing buffered data. This ensures that the \"slow\" file system is not accessed too often."
    # "Create directory if doesnt exist"
    # "File access loop (non RT loop, read from RT buffer)"
    n398 = Wait (ms)(milliseconds to wait=u32 200) -> ()  [unwired: 1 out]
    n399 = shared-variable ".\\SharedVars.lvlib\\WriteData"() -> (w972:bool)  [unwired: 1 in, 1 out]
    n400 = call "CheckFileWriteStatus-v1.vi"("WriteDataButtonVal"=w972, "WritePrevVal"=w982, "Refnum in"=w976, "Base filename"="Base filename", "File path"=path "C:/focal-data") -> ("File Name"=→"Output file Name":string, "Refnum out"=w975:refnum<k34>, "WriteCurrentVal"=w981:bool)  [unwired: 4 in]
    n401 = call "WriteToFile-v3.vi"("Refnum in"=w975, "Group Name"=w978, "IO Names"=w971, "rt fifo"=w979, "Write?"=w972, "error in (no error)"=w983, "ConstNames"=w970, "ConstValues"=w969) -> ("Writing to file"=→"Writing":bool, "error out"=w984:errorcluster)  [unwired: 5 in, 1 out]
    n402 = shared-variable ".\\SharedVars.lvlib\\StopLabVIEW"() -> (w987:bool)  [unwired: 1 in, 1 out]
    n403 = Or(x=w984, y=w987) -> (x .or. y?=w986:bool)
  }
  n404 = node-c288(w86) -> ()  [unwired: 1 out]
  n405 = node-c288(w11) -> ()  [unwired: 1 out]
  n406 = node-c288(w90) -> ()  [unwired: 1 out]
  n407 = node-c288(w25) -> ()  [unwired: 1 out]
  n408 = node-c288(w70) -> ()  [unwired: 1 out]
  n409 = node-c288(w79) -> ()  [unwired: 1 out]
  n410 = call <vilib>:"Simple Error Handler.vi"("error in (no error)"=w77) -> ()  [unwired: 4 in, 5 out]
  n411 = call <vilib>:"Simple Error Handler.vi"("error in (no error)"=w93) -> ()  [unwired: 4 in, 5 out]
